vi "Cued Discrmination Tasks w PCO (Most Recent).vi"() -> ()   [LabVIEW 2015]
uses:
  <vilib>/Utility/error.llb/DialogType.ctl
  <vilib>/Platform/TimedLoop/XDataNode/timing_clust.ctl
  <vilib>/Platform/TimedLoop/XDataNode/nitl_modes.ctl
  <vilib>/Platform/TimedLoop/XDataNode/wakeup.ctl
  <vilib>/DAQmx/read.llb/DAQmx Read (Analog 1D DBL 1Chan NSamp).vi
  <vilib>/DAQmx/read.llb/DAQmx Read (Digital Wfm 1Chan NSamp).vi
  <vilib>/DAQmx/read.llb/DAQmx Read (Counter DBL 1Chan 1Samp).vi
  <vilib>/DAQmx/write.llb/DAQmx Write (Digital Bool 1Line 1Point).vi
  <vilib>/DAQmx/write.llb/DAQmx Write (Analog 2D DBL NChan NSamp).vi
  <vilib>/DAQmx/miscellaneous.llb/DAQmx Fill In Error Info.vi
  <vilib>/platform/TimedLoop/XDataNode/XDataNode.xnode
  <vilib>/Platform/TimedLoop/XDataNode/XDNodeRunTimeDep.lvlib
panel:
  out "Stim 2":i32
  out "False Alarm":bool
  out "Diag Start Time":u32
  out "Licked":bool
  out "Reward Start (ms) \n(Discrim Vary) 2":u32
  out "Stim Start Dist \n(Discrim Vary) 2":sgl
  out "Stim Start Time\n(Discrim Vary)  2":u32
  out "Stim\nReceived 2":bool
  out "Stim\nReceived":bool
  out "Stim":i32
  out "StimInfo":i32[](array[numeric])
  out "Vert\nVariant":bool=TRUE
  out "Small Stim":bool=TRUE
  out "Numeric":i32
  out "Stim Start Dist \n(Cue Only)":sgl
  out "Stim Start Time\n(Cue Only)":u32
  out "Reward Start (ms) \n(Cue Only)":u32
  out "Stim Start Time\n(Discrim Vary)":u32
  out "Stim Start Time\n(Discrim Only)":u32
  out "Stim Variation":i16
  out "Unity Info Q":refnum<queue>
  out "Unity Version Q":refnum<queue>
  out "Stim Start Dist \n(Discrim Vary)":sgl
  out "Lick Begin \n- RZ One  2":bool=TRUE
  out "Reward Start (ms) \n(Discrim Vary)":u32
  out "Varied Stim":string
  in  "Test Encoder Speed \n(Timed Loop Period)":i64=15
  in  "Test Encoder":bool
  out "Stim Identity":string
  out "Rand Number Created":bool=TRUE
  out "UDP test":i32
  out "Unity Stim Q":refnum<queue>
  in  "Stop Unity Receive":bool
  out "UDP error":errorcluster
  out "Total Dist Travelled":dbl
  out "Reward Start (ms) \n(Discrim Only)":u32
  out "Lick Begin \n- RZ One":bool=TRUE
  out "Stim Start Dist\n(Discrim Only)":sgl
  in  "Reward Zone Finish":sgl=70.0
  in  "Reward Zone Start":sgl=30.0
  out "Encoder Ref Out":refnum<file>
  out "Encoder Ref Error":errorcluster
  out "Timer Q Out":refnum<queue>
  out "Elapsed Time":dbl caption="Elapsed Time (s)"
  out "Encoder\n Ref Out 2":refnum<file>
  out "PCo Ref Error":errorcluster
  out "File Iterations":i32
  out "Save Start Time":dbl
  out "Save Time Start":bool=TRUE
  in  "Ignore PCO":bool=TRUE
  in  "SAVE":bool
  out "Reward Start (ms) - \nRun Train":u32
  in  "Droplet Duration":u32=150
  out "Lick Waveform":i16(graph)
  out "Correct":bool
  in  "Give Soymilk":bool
  in  "Distance \nTriggered":bool
  in  "Lick Window(ms)":u32=800
  out "File Save Path":path
  in  "MODE":T1(ring)
  in  "Reward\n Distance":dbl
  in  "Rand Stim\nDist Interval":dbl=150.0 format="%#_13g"
  in  "Stop Encoder":bool
  out "Relative \nRand Dist":dbl
  in  "Hot Pixel Corr":bool
  in  "Noise Filter":bool
  in  "Mouse Name":string
  out "Red Waveform":dbl(graph)
  in  "Stop Red Stamp":bool
  out "Red Q Out":refnum<queue>
  in  "NewTrial":bool
  out "Stim ref out 2":refnum<file>
  out "Eye Track Info":sgl[](array[numeric])
  out "Eye Track Q":refnum<queue>
  out "Eye It Q":refnum<queue>
  in  "Stop Eye Cam UDP":bool
  out "Eye Iterations":u32
  out "PCO iterations":u32
  in  "Close Trigger 2":bool
  in  "Port":u16=6342
  out "bClose":bool
  in  "TriggerMode":u16(ring)=2 items=["Auto", "Software", "External sequence start ", "External exposure control"]
  in  "Delay":u32
  in  "ExposureTimeBase":u16(ring)=2 items=["nanoseconds", "microseconds", "milliseconds"]
  in  "DelayTimeBase":u16(ring)=2 items=["nanoseconds", "microseconds", "milliseconds"]
  in  "ROIX0":u16=961 min=1
  in  "ROIY0":u16=811 min=1
  out "PCO Image":u16[][](graph)
  out "PCO Ref Out 2":refnum<file>
  out "bUseBuffer0":bool
  out "bUseBuffer1":bool
  in  "Pixel Rate":i32(ring) items=["286000000", "0", "0", "0"]
  in  "Exposure":dbl=50.0
  in  "ROIX1":u16=1600
  in  "ROIY1":u16=1350
  in  "UseAcquireEnable":bool
  out "PCO Recording":bool
  in  "Close PCO":bool
  out "Bits/pixel":u16
  out "BufNr1":i16
  out "BufNr0":i16
  out "Stim ref out":refnum<file>
  out "seed 7":dbl=74805.0
  in  "xcenter 10":i32=1800
  in  "xcenter 7":i32=1800
  out "seed 5":dbl=32848.0
  out "seed 4":dbl=8420.0
  out "seed  3":dbl=16239.0
  out "seed  1":dbl=85122.0
  in  "Start Stimulus":bool
  in  "Stop TCP Write":bool
  in  "frames to avg":i32=20
  in  "Tab Control":T2(tab)=enum."akmovingspotsII"
  in  "Stimlength (s)":dbl=1.0
  in  "Scaling factor":dbl=1.0
  in  "Rects per width":dbl=320.0
  in  "Rects per height":dbl=1.0
  in  "radius":dbl=4.0
  in  "interval (s)":dbl=0.5
  in  "# of circles":dbl=10.0
  in  "# of flashes/circles":dbl=10.0
  in  "ring width":dbl=4.0
  in  "interval 2 (ms)":dbl=500.0
  in  "# of flashes/ring":dbl=2.0
  in  "spot intensity":dbl=255.0
  in  "Velocity (pix/s)":dbl=100.0
  in  "Length (pixels)":dbl=40.0
  in  "Width (pixels)":dbl=1920.0
  in  "repeats 4":i32=4
  in  "Background\nangle":dbl
  in  "Background\ncycles/s":dbl=1.0
  in  "Background\nspatial frequency":dbl=0.05
  in  "Differential time":i32=2
  in  "Local time":i32=2
  in  "Global time":i32=2
  in  "Object angle":i32=180
  in  "Object size":i32=100
  in  "Object phase":dbl
  in  "radius 2":dbl=50.0
  in  "time interval (ms)":dbl=500.0
  in  "# of x spots":dbl=2.0
  in  "# of y spots":i32=2
  in  "# of flashes/spot":i32=1
  in  "repeats 9":i32=2
  in  "flash frame length 2":i32=8
  in  "# of flashes 2":i32=8
  in  "repeats 2":dbl
  in  "y velocity":dbl
  in  "x velocity":dbl
  in  "line width":dbl
  in  "cycles per second":i32=2
  in  "period":i32=200
  in  "duration":i32=8
  in  "repeats":i32=3
  in  "amplitude":i32=100
  in  "amplitude 3":i32=100
  in  "repeats 13":i32=3
  in  "duration 3":i32=6
  in  "period 3":i32=240
  in  "cycles per second 3":i32=2
  out "seed 2":dbl=28230.0
  in  "# of flashes":i32=8
  in  "flash frame length":i32=8
  in  "repeats  11":i32=3
  in  "flashnum":i32=1
  in  "msinterval 4":i32=500
  in  "chopy":i32=5
  in  "chopx":i32=5
  in  "grayframes":i32=30
  in  "flashbrightness":i32
  in  "boxsize":i32
  in  "xcenter 4":i32
  in  "ycenter 4":i32
  in  "ycenter 6":i32
  in  "xcenter 6":i32
  in  "boxsize 2":i32
  in  "flashbrightness 2":i32
  in  "grayframes 2":i32=30
  in  "repeats  12":i32=4
  in  "flashnum 2":i32=1
  in  "msinterval 5":i32=500
  in  "chopy 2":i32=10
  in  "chopx 2":i32=10
  in  "length":i32=40
  in  "pixels/frame":i32=4
  in  "width":i32=1960
  in  "repeats 11":i32=3
  in  "bardiv":i32=1
  in  "backg 2":i32=127
  in  "barbrightness":i32
  out "seed":dbl=11328.0
  in  "0 for 90, 1 for 45":i32
  in  "graydelayframes":i32=120
  in  "RFcentered=1":i32
  in  "xcenter 5":i32
  in  "ycenter 5":i32
  in  "ycenter 8":i32
  in  "xcenter 8":i32
  in  "RFcentered=1 2":i32
  in  "graydelayframes 3":i32=120
  in  "0 for 90, 1 for 46":i32=1
  out "seed  6":dbl=32848.0
  in  "barbrightness 3":i32
  in  "backg 4":i32=127
  in  "bardiv 3":i32=1
  in  "repeats 16":i32=25
  in  "width 3":i32=1960
  in  "length 3":i32=40
  in  "pixels/frame 3":i32=4
  in  "grayframes 3":dbl=10.0
  in  "repeats 17":dbl=10.0
  in  "width 4":dbl=40.0
  in  "bars":dbl=4.0
  in  "grayframes  4":dbl=240.0
  in  "repeats  19":dbl=8.0
  in  "width  5":dbl=40.0
  in  "bars  2":dbl=6.0
  in  "grayframes  5":dbl=240.0
  in  "repeats  20":dbl=8.0
  in  "width  6":dbl=40.0
  in  "bars  3":dbl=6.0
  in  "appatchsizelitude 6":i32=300
  in  "ycenter 7":i32=500
  in  "xcenter 9":i32=1500
  in  "amplitude 5":i32=100
  in  "repeats 15":i32=10
  in  "duration 6":i32=1
  in  "period 5":i32=300
  in  "cycles per second 5":i32=1
  out "seed 6":dbl=32105.0
  in  "asdf":i32=100
  in  "asdf 2":i32=3
  in  "numpatches":i32=5
  in  "amplitude 6":i32=100
  in  "repeats 19":i32=3
  in  "duration 7":i32=5
  in  "period 6":i32=80
  in  "cycles per second 6":i32=3
  out "randinput 5":dbl=10207.0
  in  "blanktime 2":dbl=8000.0
  in  "0 for bar \n1 for cross":dbl
  in  "backg 5":dbl=127.0
  in  "centery 2":dbl=650.0
  in  "centerx 2":dbl=1500.0
  in  "repeats 18":dbl=20.0
  in  "msinterval 6":dbl=12000.0
  in  "speed 2":dbl=1.0
  in  "bar radius":dbl=1500.0
  in  "graydelayframes 2":i32
  in  "degrees":i32
  out "seed  4":dbl=22949.0
  in  "barbrightness 2":i32
  in  "backg 3":i32=127
  in  "bardiv 2":i32=1
  in  "repeats 12":i32=2
  in  "width 2":i32=1960
  in  "length 2":i32=40
  in  "pixels/frame 2":i32=4
  out "randinput 2":dbl=74805.0
  in  "grayDelay":dbl=1000.0
  in  "msinterval 2":dbl=1000.0
  in  "msDelay":dbl=1000.0
  in  "initRadius":dbl=25.0
  in  "rate":dbl=4.0
  in  "repeats 6":dbl=1.0
  in  "ycenter 2":dbl=500.0
  in  "xcenter 2":dbl=1500.0
  out "randinput 4":dbl=28230.0
  in  "grayDelay 2":dbl=1000.0
  in  "msinterval 3":dbl=1000.0
  in  "msDelay 2":dbl=1000.0
  in  "initRadius 2":dbl=25.0
  in  "rate 2":dbl=4.0
  in  "repeats 10":dbl=1.0
  in  "ycenter 3":dbl=500.0
  in  "xcenter 3":dbl=1500.0
  in  "dycenter":dbl=1000.0
  in  "dxcenter":dbl=1000.0
  in  "offsetms":dbl=1000.0
  in  "backg":dbl=127.0
  in  "centery":dbl=500.0
  in  "centerx":dbl=1700.0
  in  "repeats 3":dbl=4.0
  in  "msinterval":dbl=1000.0
  in  "speed":dbl=10.0
  in  "ringR":dbl=4.0
  in  "bool":dbl=1.0
  in  "blanktime":dbl=6000.0
  out "randinput":dbl=12910.0
  in  "background 2":i32=127
  in  "ycenter":i32=500
  in  "radius 3":i32=250
  in  "rotation":i32=90
  in  "xcenter":dbl=1700.0
  in  "period in pixels":dbl=40.0
  in  "repeats 5":dbl=4.0
  in  "period 2":dbl=6000.0
  in  "increment":i32=25
  in  "duration 2":i32=6
  in  "radius 4":i32=150
  in  "repeats 7":dbl=4.0
  in  "Ycenter":dbl=500.0
  in  "Xcenter":dbl=1700.0
  in  "gridsize":i32=4
  in  "duration 4":dbl=2.0
  in  "repeats 8":dbl=5.0
  in  "1on 2off 3 onoff":dbl=1.0
  out "randinput 3":dbl=52142.0
  in  "spotsperflash":i32=2
  out "seed 3":dbl=74805.0
  in  "amplitude 4":i32=100
  in  "repeats 14":i32=3
  in  "duration 5":i32=5
  in  "period 4":i32=80
  in  "cycles per second 4":i32=3
  in  "Frequency":i32=3
  in  "Repeats":i32=80
  in  "startCue":i32=5
  in  "waitForDeviceStart":i32=5
  in  "beepLengthSecs":i32=5
  in  "beepPauseTime":i32=5
  in  "Frequency 2":i32=3
  in  "Repeats 2":i32=80
  in  "Loops":i32=5
  in  "beepLengthSecs 2":i32=5
  in  "beepPauseTime 2":i32=5
  in  "waitForDeviceStart  2":i32=5
  in  "startCue 2":i32=5
  out "Input Line":string="34 6 40 8 120 32848 200000 10000 -330795 -230833 1869660"
  out "TCP Loop\nRunning":bool
  out "TCP Listen\nStopped":bool
  out "yref":sgl=2.9999416
  out "xref":sgl=2.9999416
  out "zref":sgl=2.9999416
  out "number (0 to 1) 2":dbl=0.7615508373602138
  out "x position":sgl=-0.30801073
  out "y position":sgl=0.69161034
  out "z position":sgl=21.696537
  out "File Open":bool
  out "PCO ref out":refnum<file>
  in  "Close Save":bool
  # "For MultAlt audio pause time starts after first crinkle -- increase if needed"
  # "Cant have less than 40"
  # "Make sure File Open &\nSave All are OFF\n when starting the VI"
  # "Set to 15 during trials"
  # "Start Flea  --> Record PCO --> Start Scanbox or Unity --> Save Flea --> Save All --> Start Stim -- > Stop Save --> New Trial ON/OFF --> Start Save --> Start Stim"
  # "Set to \"External \nSequence Start\""
  # "set to 50"
  # "Rolling       Global \n\nROIX0            1               961      \nROIX1          650            1600\n\nROIY0            1                811\nROIY1          540             1350"
  # "leave \nunselected"
  # "Global\n                       Waveform\nExp.               FR         Trig Freq\n\n50      ms       10             20           \n40.36 ms       20             20\n33.3046 ms   30                      \n500 us         33.6 \n(min. exposure time)"
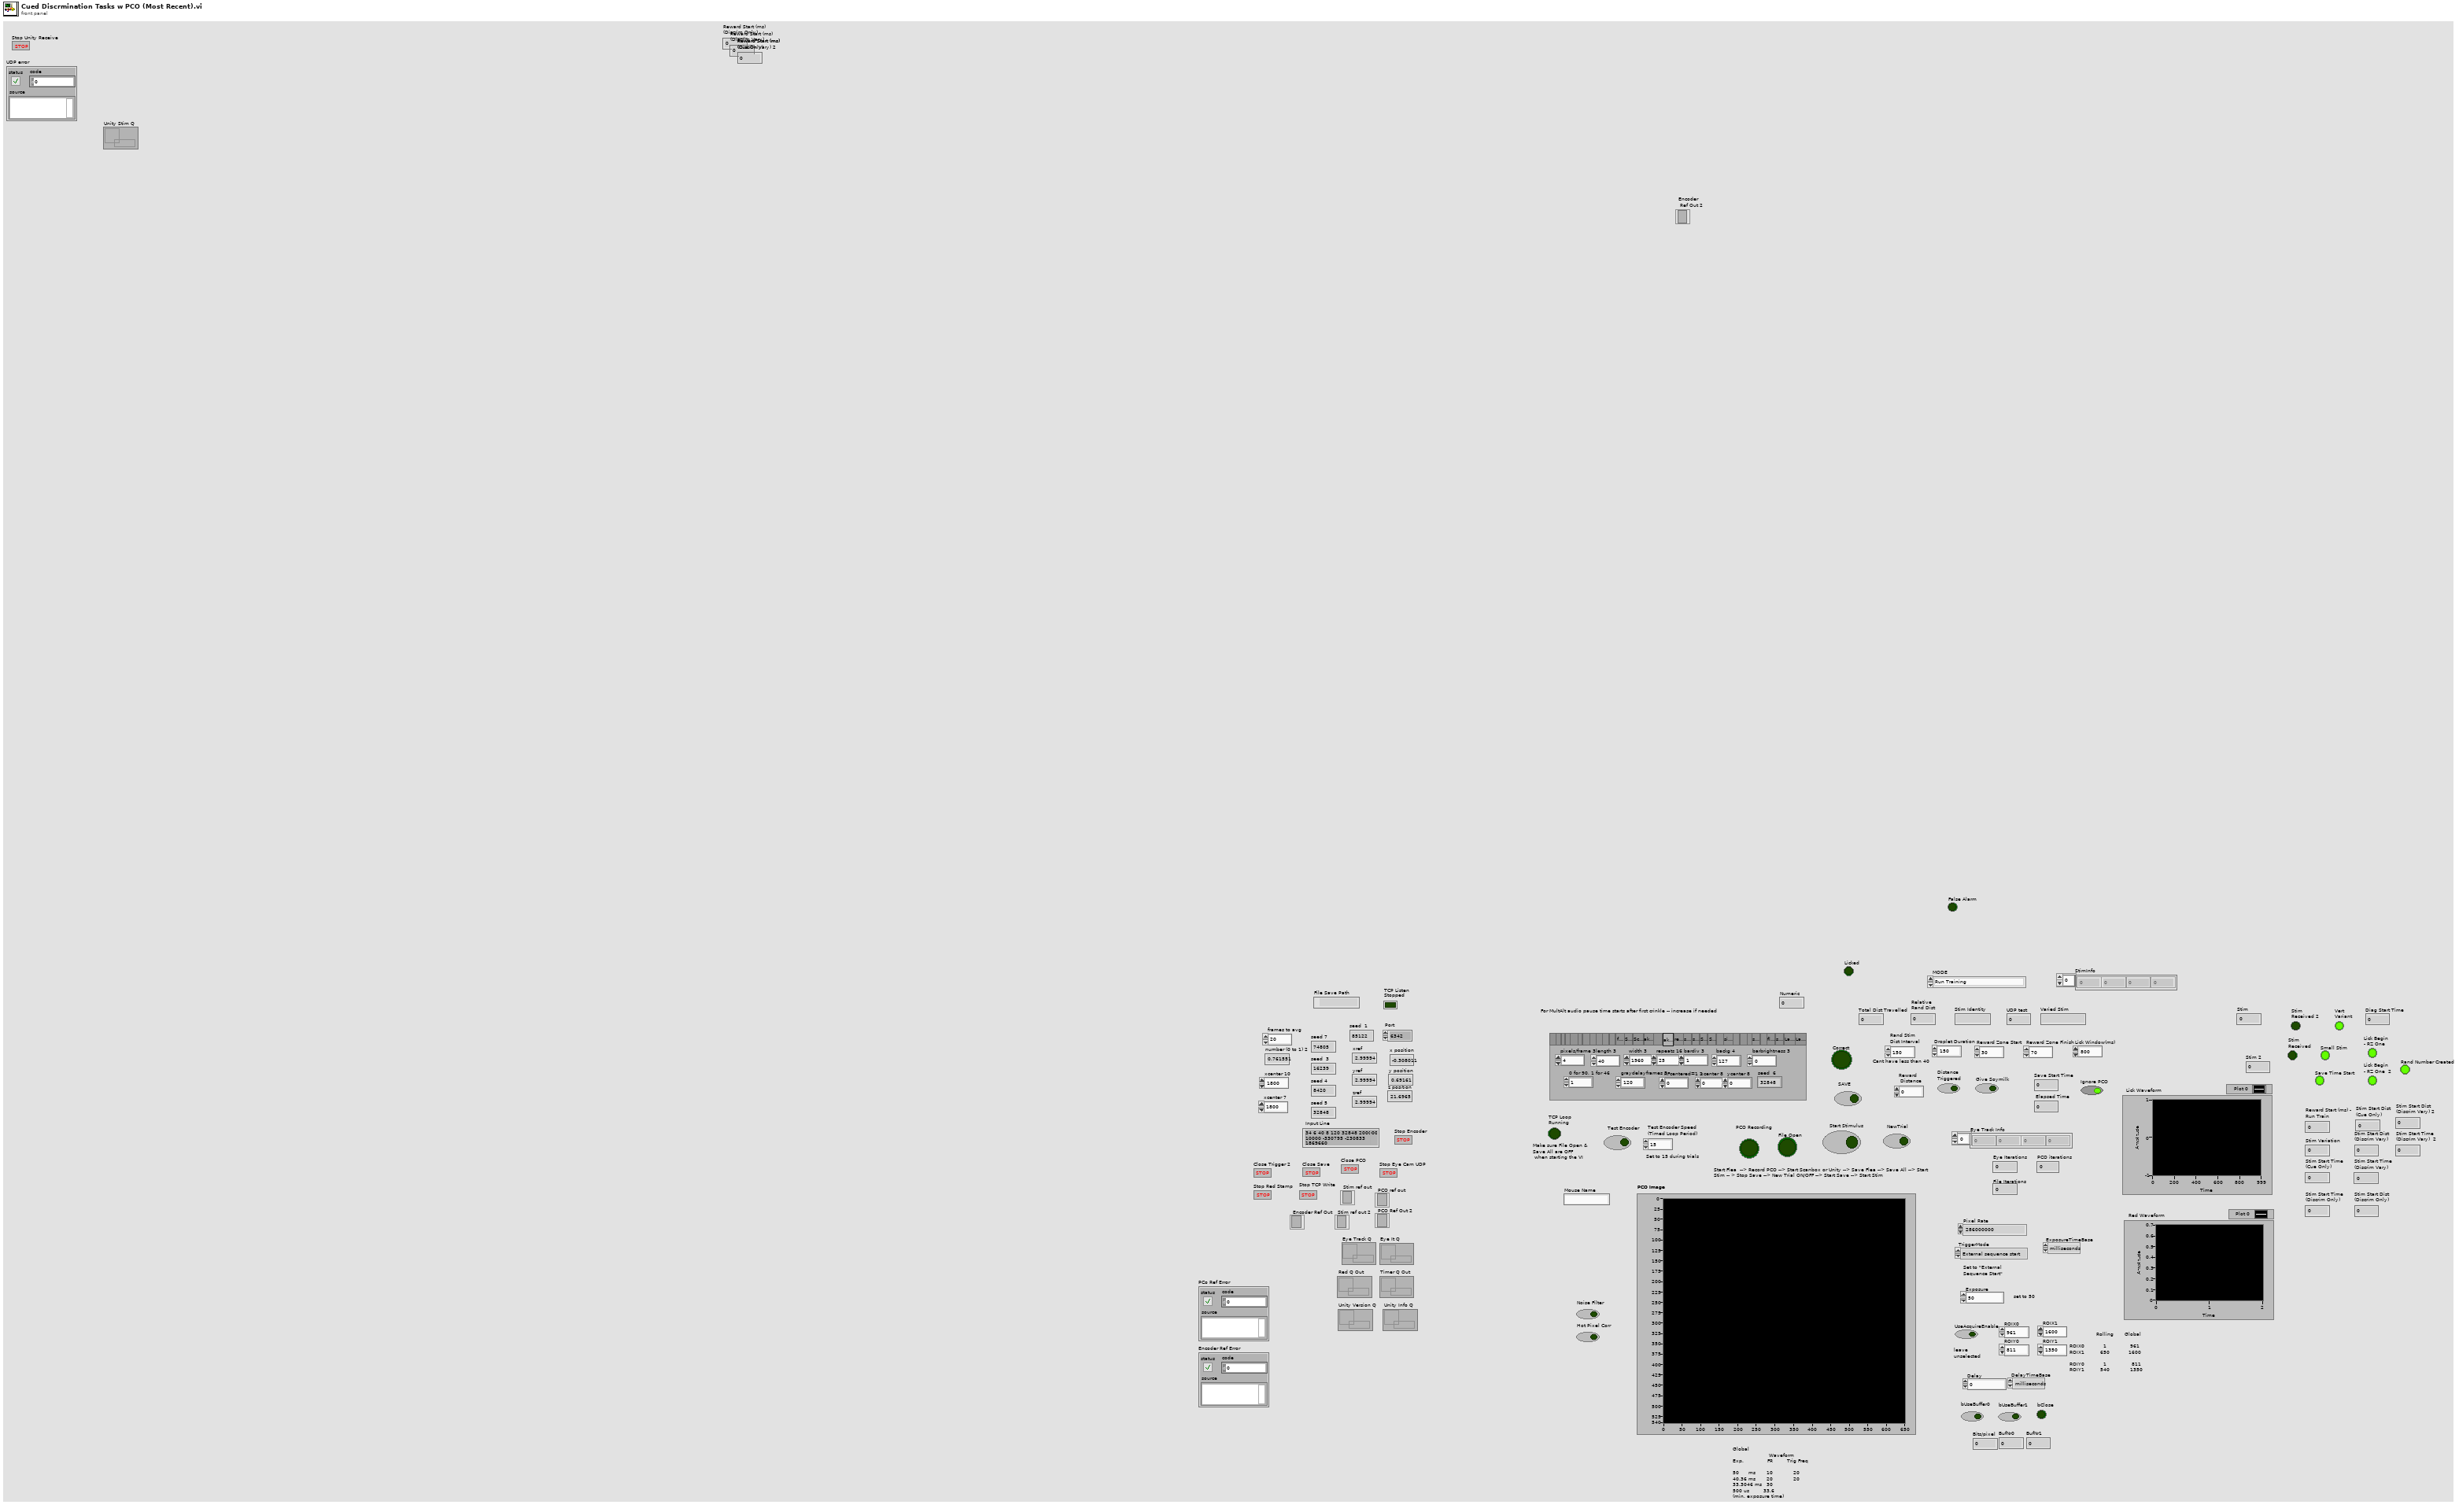
[diagram p1: front panel]
types:
  T1 = enum16{"Run Training", "Discrimination Only Task", "Discrimination Variant Task", "Alternating Variant Presentation", "Cued Attention Task "}
  T2 = enum32{"Barnoise", "Circle", "Ring", "Probe", "Moving bar", "OMS", "Rasterspot", "Fullfield", "whitebar", "driftgrat", "randgrat", "fullfieldonoff", "Screenchop", "Screenchopbars", "akmovingspots", "movingSpots", "akmovingspotsII", "retinotopybars", "slitGrtRand", "slitGrtOrder", "SqrGrtPtch", "SqrGrtPtch 2", "pinwheel", "singledirection", "newloom", "distractor", "loom", "switchgrate", "spotramp", "flickerspots", "squarewave", "LatCrinkleOneAlt", "LatCrinkleMultAlt"}
  T3 = typedef "DialogType.ctl" = u16
  T4 = cluster{"Size":u16, "CamType":u16, "CamSubType":u16, "SerialNumber":u32, "HWVersion":u32, "FWVersion":u32, "InterfaceType":u16, "HardwareVersion":cluster{"BoardNum":u16, "HWVersions":cluster{"BoardName":string, "BatchNumber":u16, "MinorRevision":u8, "MajorRevision":u8, "Variant":u16}[]}, "FirmwareVersion":cluster{"DeviceNum":u16, "FWVersions":cluster{"DeviceName":string, "MinorRevision":u8, "MajorRevision":u8, "Variant":u16}[]}}
  T5 = cluster{"Size":u16, "SensorTypeDESC":u16, "SensorSubtypeDESC":u16, "MaxHorizontalResStdDESC":u16, "MaxVerticalResStdDESC":u16, "MaxHorizontalResExtDESC":u16, "MaxVerticalResExtDESC":u16, "DynResDESC":u16, "MaxBinHorzDESC":u16, "BinHorzStepDESC":bool, "MaxBinVertDESC":u16, "BinVertStepDESC":bool, "ROIHorzStepDESC":u16, "ROIVertStepDESC":u16, "NumADCDESC":u16, "IRDESC":bool, "MinDelayDESC":u32, "MaxDelayDESC":u32, "MinDelayStepDESC":u32, "MinExpoDESC":u32, "MaxExpoDESC":u32, "MinExpoStepDESC":u32, "MinDelayIRDESC":u32, "MaxDelayIRDESC":u32, "MinExpoIRDESC":u32, "MaxExpoIRDESC":u32, "TimeTableDESC":bool, "DoubleImageDESC":bool, "MinCoolSetDESC":i16, "MaxCoolSetDESC":i16, "MDefaultCoolSetDESC":i16, "PowerDownModeDESC":bool, "OffsetRegDESC":bool, "ColorPattern":cluster{"UpperLeftColor":u8, "UpperRightColor":u8, "LowerLeftColor":u8, "LowerRightColor":u8}, "PatternTypeDESC":bool, "PixelRates":u32[], "CoversionFactors":u16[], "Reserved":u32[], "NoiseFilterCapable":bool, "HotPixelCapable":bool, "HotPixelWithNoiseFilter":bool, "ASCIITimeCapable":bool, "Extended Description":bool, "Get Extended":bool, "Reserved Flag 1":bool, "Reserved Flag 2":bool}
  T6 = typedef "XDNodeRunTimeDep.lvlib/timing_clust.ctl" = cluster{"Expected End [f-1]":u64, "Actual End [f-1]":u64, "Finished Late? [f-1]":bool, "Expected End [i-1]":u64, "Actual End [i-1]":u64, "Finished Late? [i-1]":bool, "Expected Start [i]":u64, "Actual Start [i]":u64, "Expected Start [f]":u64, "Actual Start [f]":u64, "Source Name":string, "Structure Name":string, "Period":i64, "Deadline":i64, "Offset":i64, "Start":i64, "Priority":i32, "Timeout":i32, "Mode":T7, "Wakeup Reason":T8, "Error":errorcluster, "Source Type":string, "Secondary Source Type":string, "Global End Time":u64, "Global Start Time":u64, "Frame Duration":u64, "Iteration Duration":u64, "Assigned CPU":i32, "I/O Scan Engine Mode":u32}
  T7 = typedef "XDNodeRunTimeDep.lvlib/nitl_modes.ctl" = enum32{"No Change", "Process missed periods, maintain original phase", "Discard missed periods, maintain original phase", "Process missed periods, ignore original phase", "Discard missed periods, ignore original phase"}
  T8 = typedef "XDNodeRunTimeDep.lvlib/wakeup.ctl" = enum32{"Normal", "Aborted", "Asynchronous wakeup", "Timing source error", "Timed loop error", "Timeout"}
  T9 = enum16{"open", "replace", "create", "open or create", "replace or create", "replace or create with confirmation"}
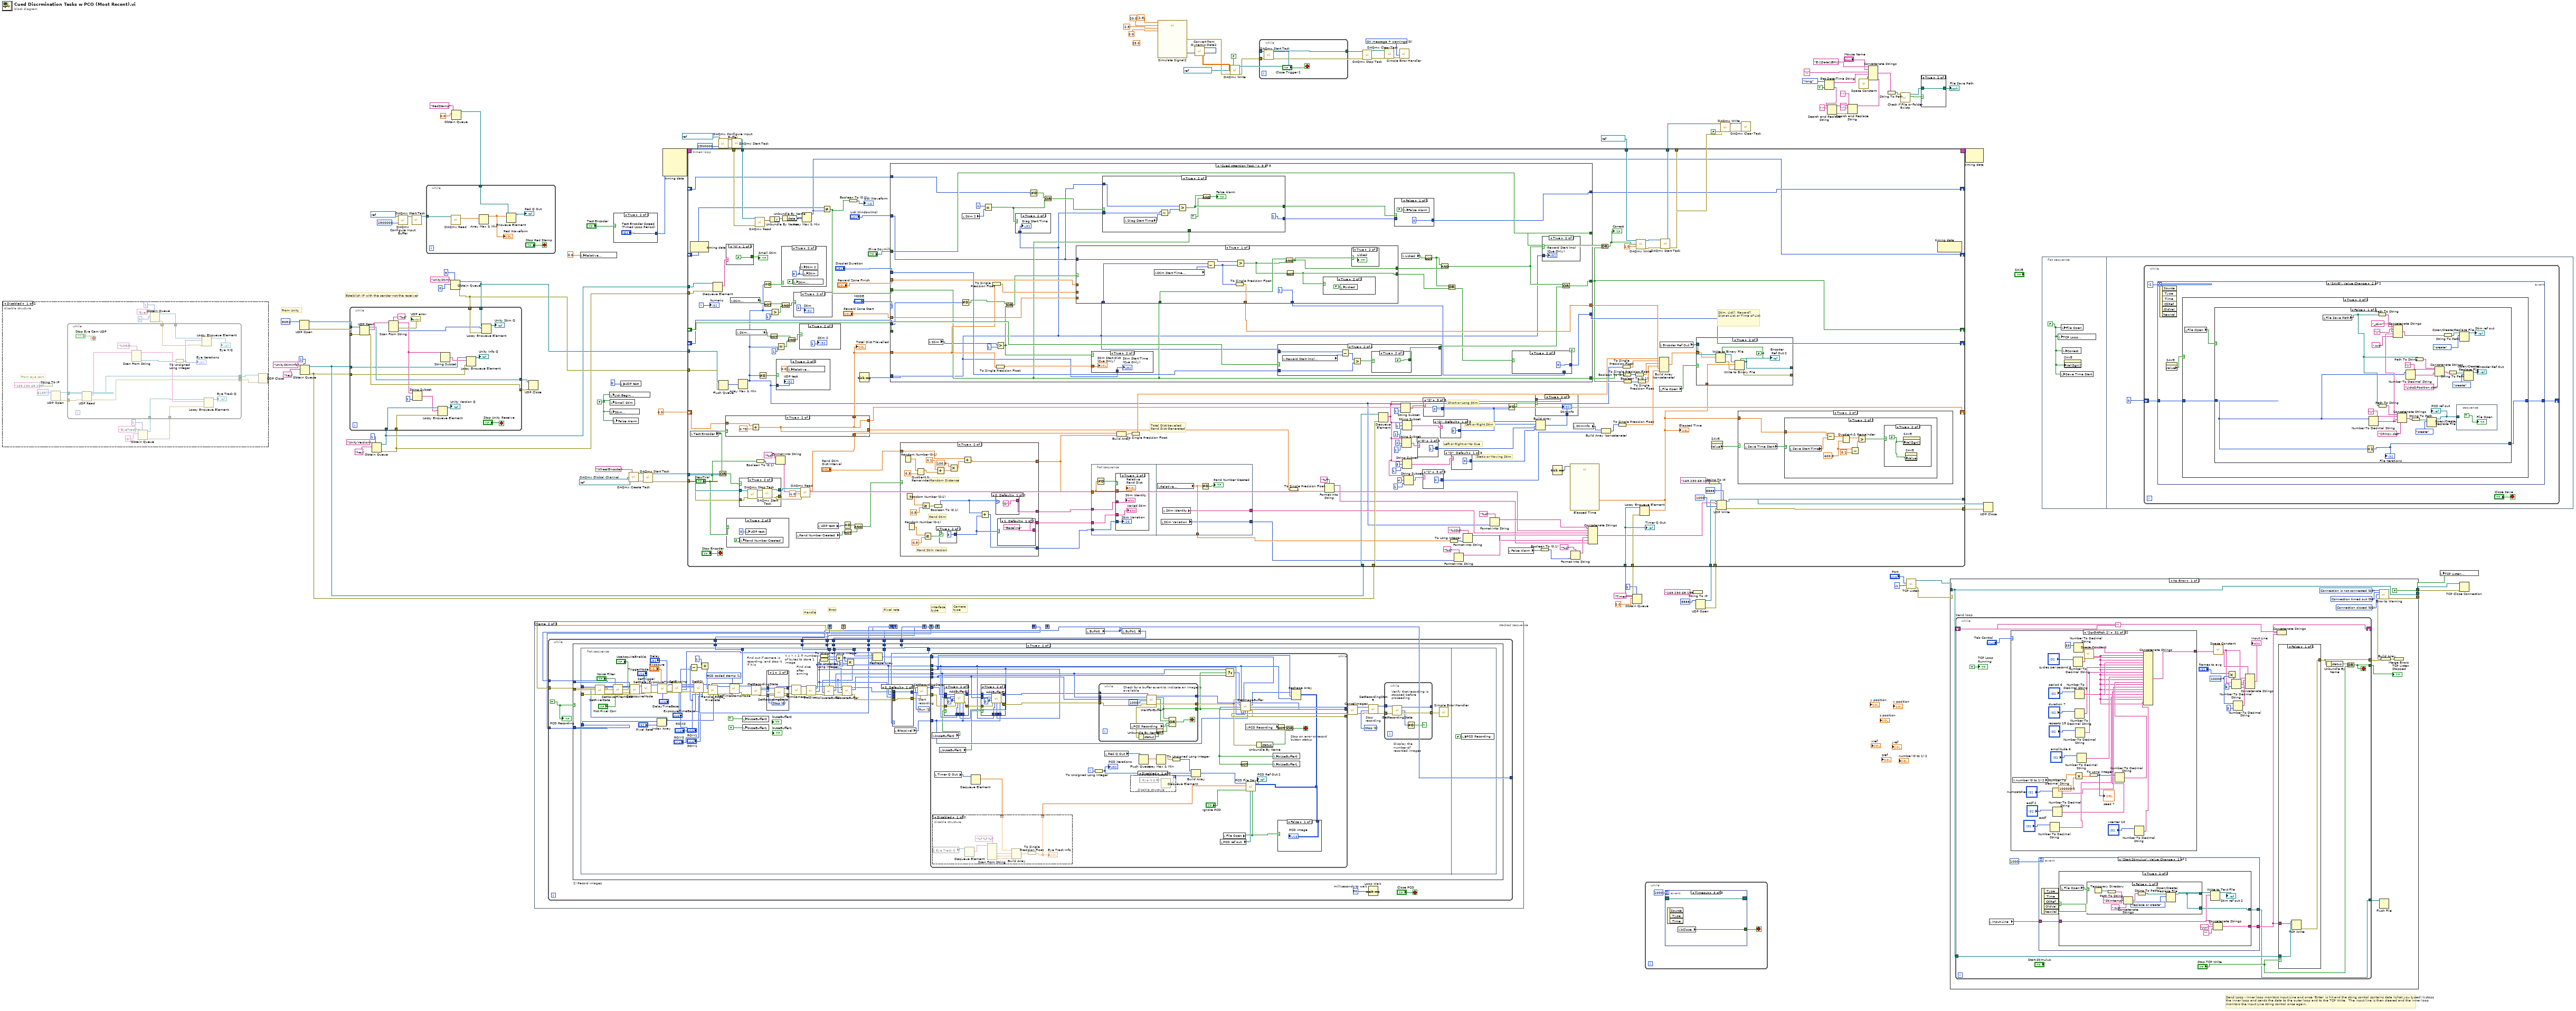
[diagram p0: block diagram]
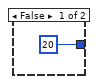
[diagram p3: hidden frame]
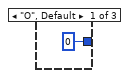
[diagram p4: hidden frame]
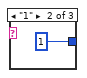
[diagram p5: hidden frame]
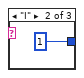
[diagram p10: hidden frame]
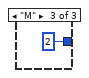
[diagram p11: hidden frame]
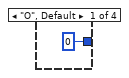
[diagram p12: hidden frame]
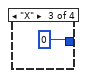
[diagram p13: hidden frame]
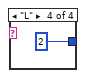
[diagram p14: hidden frame]
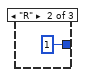
[diagram p15: hidden frame]
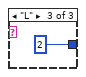
[diagram p16: hidden frame]
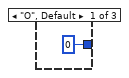
[diagram p17: hidden frame]
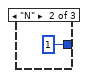
[diagram p18: hidden frame]
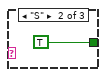
[diagram p19: hidden frame]
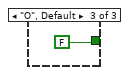
[diagram p20: hidden frame]
diagram:
  w1 = FALSE ("Lick Begin")
  w80 = refnum<k21> "MyLinearPositionChannel"  # DAQmx Global Channel
  (unwired) 25.0 ("Duty Cycle (%)")
  w97 = T3 3 items=["no dialog", "OK message", "continue or stop message", "OK message + warnings", "continue/stop + warnings"] ("type of dialog (OK msg:1)")
  # "From Unity"
  # "Establish IP with the sender not the receiver"
  # "Send Loop - Inner loop monitors Input Line and once 'Enter' is hit and the string control contains data (what you typed) it stops the inner loop and sends the data to the outer loop and to the TCP Write.  The input line is then cleared and the inner loop monitors the Input Line string control once again."
  # "Camera type"
  # "Interface type"
  # "Error"
  # "Handle"
  # "Pixel rate"
  n1 = disable-structure shown="Disabled" {
    frame Disabled {
      # "From eye cam"
      n2 = String To IP(1:"169.230.68.201" ("name")) -> ()  [unwired: 1 out]
      n3 = UDP Open(11:u16 61557 ("port")) -> (port=w121:refnum<k16>, 0:w118:errorcluster)  [unwired: 4 in, 1 out]
      n4 = Obtain Queue(max queue size (-1, unlimited)=1, name (unnamed)="EyeTrack", element data type="0" ("format string")) -> (queue out=w109:refnum<queue>, error out=w108:errorcluster)  [unwired: 2 in, 1 out]
      n5 = Obtain Queue(max queue size (-1, unlimited)=1, name (unnamed)="EyeIt", element data type=u32 0 ("Eye Iterations")) -> (queue out=w114:refnum<queue>, error out=w113:errorcluster)  [unwired: 2 in, 1 out]
      n6 = while {
        tunnel: w121 -> [w137]
        tunnel: [w135] -> w122
        tunnel: w118 -> [w136]
        tunnel: [w134] -> w123
        tunnel: w114 -> [w127]
        tunnel: w113 -> [w126]
        tunnel: w109 -> [w125]
        tunnel: w108 -> [w124]
        stop <- "Stop Eye Cam UDP" stop-if-true
        n7 = UDP Read(connection ID=w137, 8:w136) -> (data out=w129:string, error out=w134:errorcluster, 3:w135:refnum<k16>)  [unwired: 2 in, 2 out]
        n8 = Scan From String(format string="%05d", input string=w129) -> (remaining string=w128:string, output 1=w139:i32)  [unwired: 3 in, 2 out]
        n9 = To Unsigned Long Integer(number=w139) -> (unsigned 32bit integer=w133:u32)
        "Eye Iterations" <- w133
        n10 = Lossy Enqueue Element(queue=w127, element=w133, error in (no error)=w126) -> (queue out=→"Eye It Q":refnum<queue>)  [unwired: 3 out]
        n11 = Lossy Enqueue Element(queue=w125, element=w128, error in (no error)=w124) -> (queue out=→"Eye Track Q":refnum<queue>)  [unwired: 3 out]
      }
      n12 = UDP Close(connection ID=w122, 8:w123) -> ()  [unwired: 2 out]
    }
    frame Enabled {
    }
  }
  n13 = UDP Open(11:u16 8051 ("port")) -> (port=w24:refnum<k16>, 0:w23:errorcluster)  [unwired: 4 in, 1 out]
  n14 = Obtain Queue(max queue size (-1, unlimited)=1, name (unnamed)="UnityStimInfo", element data type="hey") -> (queue out=w4:refnum<queue>, error out=w3:errorcluster)  [unwired: 2 in, 1 out]
  n15 = Obtain Queue(max queue size (-1, unlimited)=1, name (unnamed)="UnityVersion", element data type="hey") -> (queue out=w8:refnum<queue>, error out=w7:errorcluster)  [unwired: 2 in, 1 out]
  n16 = call <vilib>:"DAQmx Configure Input Buffer.vi"("task/channels in"=refnum<k21> "RedStamp", "buffer size (in samples per channel)"=u32 2500000) -> ("task out"=w76:refnum<k21>)  [unwired: 12 in, 1 out]
  n17 = call <vilib>:"DAQmx Start Task.vi"("task/channels in"=w76) -> ("task out"=w78:refnum<k21>)  [unwired: 13 in, 1 out]
  n18 = Obtain Queue(max queue size (-1, unlimited)=5, name (unnamed)="UnityStim", element data type=0 ("Eye Iterations")) -> (queue out=w17:refnum<queue>, error out=w16:errorcluster)  [unwired: 2 in, 1 out]
  n19 = while {
    tunnel: w24 -> [w161]
    tunnel: w23 -> [w160]
    tunnel: [w150] -> w22
    tunnel: [w158] -> w21
    tunnel: w17 -> [w156]
    tunnel: w16 -> [w155]
    tunnel: w7 -> [w148]
    tunnel: w8 -> [w149]
    tunnel: w4 -> [w141]
    tunnel: w3 -> [w140]
    stop <- "Stop Unity Receive" stop-if-true
    n20 = UDP Read(connection ID=w161, 8:w160) -> (data out=w157:string, error out=w158:errorcluster, 3:w150:refnum<k16>)  [unwired: 2 in, 2 out]
    n21 = Scan From String "Scan From String"(format string="%d", input string=w157) -> (remaining string=w144:string, error out=→"UDP error":errorcluster, output 1=w154:i32)  [unwired: 3 in, 1 out]
    n22 = String Subset(string=w144, length (rest)=1 ("length (rest)")) -> (substring=w145:string)  [unwired: 1 in]
    n23 = Lossy Enqueue Element(queue=w149, element=w145, error in (no error)=w148) -> (queue out=→"Unity Version Q":refnum<queue>)  [unwired: 3 out]
    n24 = String Subset(string=w144) -> (substring=w142:string)  [unwired: 2 in]
    n25 = Lossy Enqueue Element(queue=w141, element=w142, error in (no error)=w140) -> (queue out=→"Unity Info Q":refnum<queue>)  [unwired: 3 out]
    n26 = Lossy Enqueue Element(queue=w156, element=w154, error in (no error)=w155) -> (queue out=→"Unity Stim Q":refnum<queue>)  [unwired: 3 out]
  }
  n27 = Obtain Queue(name (unnamed)="RedStamp", element data type=0.0 ("max value")) -> (queue out=w74:refnum<queue>)  [unwired: 3 in, 2 out]
  n28 = while {
    tunnel: w78 -> [w167]
    tunnel: w74 -> [w165]
    stop <- "Stop Red Stamp" stop-if-true
    n29 = call-poly <vilib>:"DAQmx Read.vi"("task/channels in"=w167) -> ("data"=w163:dbl[])  [unwired: 12 in, 2 out]
    n30 = Array Max & Min(array=w163) -> (max value=w162:dbl)  [unwired: 3 out]
    "Red Waveform" <- w162
    n31 = Enqueue Element(queue=w165, element=w162) -> (queue out=→"Red Q Out":refnum<queue>)  [unwired: 2 in, 2 out]
  }
  n32 = UDP Close(connection ID=w22, 8:w21) -> ()  [unwired: 2 out]
  n33 = stacked-sequence {
    seq-local: [w212 _ _] -> [_ w232 _]
    seq-local: [w185 _ _] -> [_ _ _]
    seq-local: [w173 _ _] -> [_ w235 w456]
    seq-local: [w174 _ _] -> [_ w234 w455]
    seq-local: [w210 _ _] -> [_ w233 _]
    seq-local: [w200 _ _] -> [_ w229 _]
    seq-local: [w187 _ _] -> [_ w228 _]
    seq-local: [w184 _ _] -> [_ w227 _]
    seq-local: [w183 _ _] -> [_ w226 _]
    frame #0 {
      w202 = FALSE ("stop")
      # "Setup greyscale palette for intensity graph display: Color = i*(0x01 + 0x100 + 0x10000)"
      # "1) Setup camera"
      # "Find out if camera uses CameraLink"
      # "Initialize a LabVIEW array of X x Y integers to hold image"
      # "Open communication with a camera and find its properties"
      n34 = local write "PCO Recording"(w202) -> ()
      n35 = local write "bClose"(w202) -> ()
      n36 = call <vilib>:"Reset_SDK_Lib.vi"() -> ("ErrorOut"=w168:errorcluster)  [unwired: 11 in]
      n37 = call <vilib>:"OpenCamera.vi"("ErrorIn"=w168) -> ("ErrorOut"=w198:errorcluster, "Handle out"=w199:u64)  [unwired: 3 in, 2 out]
      n38 = call <vilib>:"InitLibrary.vi"("error in (no error)"=w198, "InterfaceType"=u32 3, "ph"=w199) -> ("error out"=w197:errorcluster, "hout"=w196:u64)  [unwired: 7 in]
      n39 = for {
        N: 256 -> [_]
        tunnel: [w216] -> w178 mode=indexing
        i -> [w217]
        n40 = Multiply(x=65793, y=w217) -> (x*y=w216:i32)
      }
      n41 = call <vilib>:"GetCameraType.vi"("ph"=w196, "error in (no error)"=w197) -> ("hout"=w182:u64, "CameraType"=w188:T4, "error out"=w181:errorcluster)  [unwired: 1 in, 1 out]
      n42 = call <vilib>:"GetDescription.vi"("ErrorIn"=w181, "ph"=w182) -> ("ErrorOut"=w170:errorcluster, "Description"=w211:T5, "hout"=w172:u64)  [unwired: 2 in, 1 out]
      n43 = call <vilib>:"GetAcquireEnableSignalStatus.vi"("error in (no error)"=w170, "ph"=w172) -> ("error out"=w169:errorcluster, "hout"=w171:u64)  [unwired: 2 in, 2 out]
      n44 = Unbundle By Name(w188) -> ("InterfaceType"=w210:u16)
      n45 = Unbundle By Name(w188) -> ("CamType"=w187:u16)
      n46 = property on="PCO Image" class="IntGraph (strict)"("Y Scale.Flipped"=TRUE, "X Scale.Flipped"=FALSE, "Color Table"=w178) -> ()  [unwired: 2 in, 2 out]
      n47 = Unbundle By Name(w211) -> ("DynResDESC"=→"Bits/pixel":u16, "PixelRates"=w200:u32[], "MaxHorizontalResStdDESC"=w176:u16, "MaxVerticalResStdDESC"=w175:u16, "MaxBinHorzDESC"=w184:u16, "MaxBinVertDESC"=w183:u16)  [unwired: 4 out]
      n48 = Number To Decimal String(number=w200) -> (decimal integer string=w201:string[])  [unwired: 1 in]
      n49 = property on="Pixel Rate" class="Ring (strict)"("Strings []"=w201) -> ()  [unwired: 2 in, 2 out]
      n50 = call <vilib>:"GetRecordingState.vi"("ErrorIn"=w169, "ph"=w171) -> ("ErrorOut"=w192:errorcluster, "Error"=w186:i32, "hout"=w193:u64)  [unwired: 2 in, 1 out]
      n51 = To Unsigned Long Integer(number=w176) -> (unsigned 32bit integer=w207:u32)
      n52 = To Unsigned Long Integer(number=w175) -> (unsigned 32bit integer=w206:u32)
      n53 = case shown="0, Default" w186 {
        tunnel: w193 -> [w222 w225]
        tunnel: w192 -> [w221 w224]
        tunnel: [w220 w225] -> w191
        tunnel: [w219 w224] -> w189
        frame 0, Default {
          w223 = u16 0 items=["Stop", "Run"] ("RecordingState")
          n54 = call <vilib>:"SetRecordingState.vi"("ErrorIn"=w221, "RecordingState"=w223, "ph"=w222) -> ("ErrorOut"=w219:errorcluster, "hout"=w220:u64)  [unwired: 2 in, 1 out]
        }
        frame 1 {
        }
      }
      n55 = Multiply(x=w207, y=w206) -> (x*y=w213:u32)
      n56 = Initialize Array(u16 0 ("Element Data"), w213) -> (w212:u16[])
      n57 = Multiply(x=w213, y=u32 2) -> (x*y=w185:u32)
      n58 = call <vilib>:"AllocateBuffer.vi"("error in (no error)"=w189, "Size"=w185, "BufNr"=i16 -1, "ph"=w191) -> ("error out"=w194:errorcluster, "BufNrOut"=→"BufNr0":i16, "hout"=w190:u64)  [unwired: 2 in, 3 out]
      n59 = call <vilib>:"AllocateBuffer.vi"("error in (no error)"=w194, "BufNr"=i16 -1, "ph"=w190) -> ("error out"=w174:errorcluster, "BufNrOut"=→"BufNr1":i16, "hout"=w173:u64)  [unwired: 3 in, 3 out]
    }
    frame #1 {
      n60 = local read "BufNr0"() -> (w231:i16)
      n61 = local read "BufNr1"() -> (w230:i16)
      n62 = while {
        tunnel: w231 -> [_]
        tunnel: w231 -> [w244]
        tunnel: w232 -> [w246]
        tunnel: w233 -> [w247]
        tunnel: w234 -> [w245]
        tunnel: w235 -> [w242]
        tunnel: w230 -> [w243]
        tunnel: w229 -> [w241]
        tunnel: w228 -> [w240]
        tunnel: w227 -> [w239]
        tunnel: w226 -> [w238]
        stop <- "Close PCO" stop-if-true
        w236 = TRUE
        w248 = u32 50  # milliseconds to wait
        n63 = case "2) Record images" shown="True" w236 {
          tunnel: w242 -> [_ w258]
          tunnel: w245 -> [_ w257]
          tunnel: w247 -> [_ w256]
          tunnel: w246 -> [_ w255]
          tunnel: w244 -> [_ w254]
          tunnel: w243 -> [_ w253]
          tunnel: w241 -> [_ w252]
          tunnel: w240 -> [_ w251]
          tunnel: w239 -> [_ w250]
          tunnel: w238 -> [_ w249]
          frame False {
          }
          frame True {
            n64 = flat-sequence {
              tunnel: w258 -> [w330]
              tunnel: w257 -> [w329]
              tunnel: w256 -> [w327]
              tunnel: w255 -> [w325]
              tunnel: w254 -> [w317]
              tunnel: w253 -> [w314]
              tunnel: w252 -> [w305]
              tunnel: w251 -> [w300]
              tunnel: w250 -> [w295]
              tunnel: w249 -> [w294]
              frame #0 {
                w271 = u16 1 items=["No time stamp", "BCD coded stamp", "BCD stamp + ASCII text"] ("TimeStampMode")
                w340 = u16 1 items=["Stop", "Run"] ("RecordingState")
                w343 = u16 0 items=["Stop", "Run"] ("RecordingState")
                # "Display the number of recorded images"
                # "Start recording"
                # "Find size after arming"
                # "Find out if camera is recording, and stop it if it is"
                # "X x Y x 2 = number of bytes to store 1 image"
                # "Stop recording"
                n65 = Index Array(array=w305, index="Pixel Rate") -> (element=w304:u32)
                n66 = call <vilib>:"SetPixelRate.vi"("error in (no error)"=w329, "PixelRate"=w304, "ph"=w330) -> ("error out"=w268:errorcluster, "hout"=w270:u64)  [unwired: 2 in, 1 out]
                n67 = call <vilib>:"SetNoiseFilterMode.vi"("error in (no error)"=w268, "Hot Pixel Corr"="Hot Pixel Corr", "Noise Filter"="Noise Filter", "ph"=w270) -> ("error out"=w267:errorcluster, "hout"=w269:u64)  [unwired: 1 out]
                n68 = call <vilib>:"SetAcquireMode.vi"("error in (no error)"=w267, "UseAcquireEnable"="UseAcquireEnable", "ph"=w269) -> ("error out"=w273:errorcluster, "hout"=w274:u64)  [unwired: 2 in, 1 out]
                n69 = call <vilib>:"SetTrigger.vi"("error in (no error)"=w273, "TriggerMode"="TriggerMode", "ph"=w274) -> ("error out"=w276:errorcluster, "hout"=w275:u64)  [unwired: 2 in, 1 out]
                n70 = call <vilib>:"SetDelayExposureTime.vi"("ph"=w275, "Delay"="Delay", "Exposure"="Exposure", "error in (no error)"=w276, "DelayTimeBase"="DelayTimeBase", "ExposureTimeBase"="ExposureTimeBase") -> ("hout"=w292:u64, "error out"=w291:errorcluster)  [unwired: 7 in, 1 out]
                n71 = call <vilib>:"SetBinning.vi"("error in (no error)"=w291, "BinVert"=w294, "BinHorz"=w295, "ph"=w292) -> ("error out"=w287:errorcluster, "hout"=w289:u64)  [unwired: 3 in, 1 out]
                n72 = Subtract(x="ROIX1", y="ROIX0") -> (x-y=w303:u16)
                n73 = call <vilib>:"SetROI.vi"("ph"=w289, "ROIX0"="ROIX0", "ROIY0"="ROIY0", "ROIX1"="ROIX1", "ROIY1"="ROIY1", "error in (no error)"=w287) -> ("hout"=w288:u64, "error out"=w286:errorcluster)  [unwired: 12 in]
                n74 = Add(x=1, y=w303) -> (x+y=w301:i32)
                n75 = call <vilib>:"Handle_Edge_Pixelrate.vi"("Cameratype"=w300, "error in (no error)"=w286, "PixelRate"=w304, "X-Resolution"=w301, "ph"=w288) -> ("error out"=w263:errorcluster, "hout"=w264:u64)  [unwired: 5 in]
                n76 = call <vilib>:"SetTimeStampMode.vi"("error in (no error)"=w263, "TimeStampMode"=w271, "ph"=w264) -> ("error out"=w260:errorcluster, "hout"=w259:u64)  [unwired: 1 out]
                n77 = local write "bUseBuffer0"(TRUE) -> ()
                n78 = local write "bUseBuffer1"(TRUE) -> ()
                n79 = call <vilib>:"GetRecordingState.vi"("ErrorIn"=w260, "ph"=w259) -> ("ErrorOut"=w337:errorcluster, "RecordingState"=w339:u16, "hout"=w338:u64)  [unwired: 2 in, 1 out]
                n80 = case shown="1" w339 {
                  tunnel: w338 -> [w448 w452]
                  tunnel: w337 -> [w447 w451]
                  tunnel: [w448 w450] -> w336
                  tunnel: [w447 w449] -> w335
                  frame 0, Default {
                  }
                  frame 1 {
                    w453 = u16 0 items=["Stop", "Run"] ("RecordingState")
                    n81 = call <vilib>:"SetRecordingState.vi"("ErrorIn"=w451, "RecordingState"=w453, "ph"=w452) -> ("ErrorOut"=w449:errorcluster, "hout"=w450:u64)  [unwired: 2 in, 1 out]
                  }
                }
                n82 = call <vilib>:"ArmCamera.vi"("error in (no error)"=w335, "ph"=w336) -> ("error out"=w261:errorcluster, "hout"=w262:u64)  [unwired: 1 in, 1 out]
                n83 = call <vilib>:"GetSizes.vi"("ph"=w262, "ErrorIn"=w261) -> ("hout"=w298:u64, "XResAct"=w323:u16, "YResAct"=w322:u16, "ErrorOut"=w297:errorcluster)  [unwired: 11 in, 3 out]
                n84 = To Unsigned Long Integer(number=w323) -> (unsigned 32bit integer=w318:u32)
                n85 = To Unsigned Long Integer(number=w322) -> (unsigned 32bit integer=w319:u32)
                n86 = Multiply(x=w318, y=w319) -> (x*y=w320:u32)
                n87 = Multiply(x=w320, y=u32 2) -> (x*y=w285:u32)
                n88 = call <vilib>:"AllocateBuffer.vi"("error in (no error)"=w297, "Size"=w285, "BufNr"=w317, "ph"=w298) -> ("error out"=w316:errorcluster, "BufNrOut"=w299:i16, "hout"=w315:u64)  [unwired: 2 in, 3 out]
                n89 = call <vilib>:"AllocateBuffer.vi"("error in (no error)"=w316, "Size"=w285, "BufNr"=w314, "ph"=w315) -> ("error out"=w283:errorcluster, "BufNrOut"=w313:i16, "hout"=w284:u64)  [unwired: 2 in, 3 out]
                n90 = Reshape Array(w325, w320) -> (w324:u16[])
                n91 = case shown="0, Default" w327 {
                  tunnel: [w440 w446] -> w331
                  tunnel: w322 -> [_ w445]
                  tunnel: w323 -> [_ w444]
                  tunnel: w284 -> [w440 w443]
                  tunnel: w283 -> [w439 w442]
                  tunnel: [w439 w441] -> w296
                  frame 0, Default {
                  }
                  frame 2 {
                    # "Only necessary if the interface is Camera Link"
                    n92 = call <vilib>:"CamLinkSetImageParameters.vi"("error in (no error)"=w442, "YRes"=w445, "XRes"=w444, "ph"=w443) -> ("error out"=w441:errorcluster, "hout"=w446:u64)  [unwired: 1 out]
                  }
                }
                n93 = local read "Bits/pixel"() -> (w310:u16)
                n94 = call <vilib>:"SetRecordingState.vi"("ErrorIn"=w296, "RecordingState"=w340, "ph"=w331) -> ("ErrorOut"=w328:errorcluster, "hout"=w326:u64)  [unwired: 2 in, 1 out]
                n95 = while {
                  tunnel: w299 -> [w380]
                  tunnel: w324 -> [w364]
                  tunnel: w326 -> [w384]
                  tunnel: w322 -> [w370]
                  tunnel: w323 -> [w368]
                  tunnel: w328 -> [w382]
                  tunnel: [w366] -> w309
                  tunnel: [w365] -> w308
                  tunnel: w313 -> [w373]
                  tunnel: w310 -> [w369]
                  i -> [w374]
                  stop <- w375 stop-if-true
                  # "Stop on error or record button status"
                  n96 = local read "bUseBuffer0"() -> (w359:bool)
                  n97 = local read "Timer Q Out"() -> (w345:refnum<queue>)
                  n98 = local read "bUseBuffer1"() -> (w358:bool)
                  n99 = case shown="True" w359 {
                    tunnel: [w399 w408] -> w381
                    tunnel: [w398 w407] -> w383
                    tunnel: w380 -> [_ w406]
                    tunnel: w384 -> [w398 w405]
                    tunnel: w369 -> [_ w403]
                    tunnel: w368 -> [_ w402]
                    tunnel: w370 -> [_ w401]
                    tunnel: w382 -> [w399 w400]
                    frame False {
                    }
                    frame True {
                      w404 = i16 0
                      n100 = call <vilib>:"AddBufferEX.vi"("ph"=w405, "BuffNr"=w406, "1stImage"=w404, "LastImage"=w404, "error in (no error)"=w400, "XRes"=w402, "YRes"=w401, "BitPerPixel"=w403) -> ("hout"=w407:u64, "error out"=w408:errorcluster)  [unwired: 5 in, 1 out]
                    }
                  }
                  n101 = Dequeue Element(queue=w345) -> (element=w344:dbl)  [unwired: 2 in, 3 out]
                  n102 = disable-structure shown="Disabled" {
                    disable-tunnel: [w389 _] -> w347
                    disable-tunnel: w344 -> [w388 _]
                    frame Disabled {
                      n103 = local read "Eye Track Q"() -> (w390:refnum<queue>)
                      n104 = Dequeue Element(queue=w390) -> (element=w395:string)  [unwired: 2 in, 3 out]
                      n105 = Scan From String(format string="%f %f %f", input string=w395) -> (output 1=w394:dbl, output 2=w393:dbl, output 3=w392:dbl)  [unwired: 5 in, 3 out]
                      n106 = Build Array(w388, w394, w393, w392) -> (w391:dbl[])
                      n107 = To Single Precision Float(number=w391) -> (single precision float=w389:sgl[])
                      "Eye Track Info" <- w389
                    }
                    frame Enabled {
                    }
                  }
                  n108 = case shown="True" w358 {
                    tunnel: [w409 w419] -> w371
                    tunnel: [w410 w418] -> w372
                    tunnel: w373 -> [_ w417]
                    tunnel: w383 -> [w410 w416]
                    tunnel: w369 -> [_ w414]
                    tunnel: w368 -> [_ w413]
                    tunnel: w370 -> [_ w412]
                    tunnel: w381 -> [w409 w411]
                    frame False {
                    }
                    frame True {
                      w415 = i16 0
                      n109 = call <vilib>:"AddBufferEX.vi"("ph"=w416, "BuffNr"=w417, "1stImage"=w415, "LastImage"=w415, "error in (no error)"=w411, "XRes"=w413, "YRes"=w412, "BitPerPixel"=w414) -> ("hout"=w418:u64, "error out"=w419:errorcluster)  [unwired: 5 in, 1 out]
                    }
                  }
                  n110 = To Unsigned Long Integer(number=w374) -> (unsigned 32bit integer=w352:u32)
                  "PCO iterations" <- w352
                  n111 = while {
                    tunnel: w380 -> [w421]
                    tunnel: [w431] -> w379
                    tunnel: [w429] -> w378
                    tunnel: [w427] -> w361
                    tunnel: w372 -> [w426]
                    tunnel: w371 -> [w425]
                    tunnel: w373 -> [w420]
                    stop <- w432 stop-if-true
                    # "Check for a buffer event to indicate an image is available"
                    n112 = local read "PCO Recording"() -> (w423:bool)
                    n113 = call <vilib>:"WaitForBuffer.vi"("ph"=w426, "sBufNr"=w421, "sBufNr 2"=w420, "timeout"=1000, "error in (no error)"=w425) -> ("hout"=w431:u64, "Buffer_Ready"=w427:bool, "Buffer_Ready 2"=w422:bool, "error out"=w429:errorcluster)  [unwired: 10 in, 1 out]
                    n114 = Unbundle By Name(w429) -> ("status"=w428:bool)
                    n115 = Not(x=w428) -> (.not. x?=w424:bool)
                    n116 = Compound Arithmetic op=OR(w427, w422, w423, w424) -> (w432:bool)
                  }
                  n117 = local read "Red Q Out"() -> (w355:refnum<queue>)
                  n118 = disable-structure shown="Disabled" {
                    disable-tunnel: [w386 _] -> w348
                    frame Disabled {
                      n119 = local read "Eye It Q"() -> (w387:refnum<queue>)
                      n120 = Dequeue Element(queue=w387) -> (element=w386:u32)  [unwired: 2 in, 3 out]
                    }
                    frame Enabled {
                    }
                  }
                  n121 = Flush Queue(queue=w355) -> (remaining elements=w354:dbl[])  [unwired: 1 in, 2 out]
                  n122 = Array Max & Min(array=w354) -> (max value=w353:dbl)  [unwired: 3 out]
                  n123 = To Unsigned Long Integer(number=w353) -> (unsigned 32bit integer=w351:u32)
                  n124 = Build Array(w351, w352, w348) -> (w350:u32[])
                  n125 = local read "PCO ref out"() -> (w357:refnum<file>)
                  n126 = local read "File Open"() -> (w356:bool)
                  n127 = Select(t=w380, s=w361, f=w373) -> (s? t:f=w367:i16)
                  n128 = Not(x=w361) -> (.not. x?=w360:bool)
                  n129 = call <vilib>:"GetImageBuffer.vi"("ph"=w379, "BuffIn"=w364, "BuffNr"=w367, "error in (no error)"=w378, "xRes"=w368, "yRes"=w370, "Bitresolution"=w369) -> ("hout"=w366:u64, "BuffOut"=w363:u16[], "error out"=w365:errorcluster)  [unwired: 5 in, 1 out]
                  n130 = local read "PCO Recording"() -> (w385:bool)
                  n131 = Unbundle By Name(w378) -> ("status"=w376:bool)
                  n132 = local write "bUseBuffer0"(w361) -> ()
                  n133 = local write "bUseBuffer1"(w360) -> ()
                  n134 = Not(x=w385) -> (.not. x?=w377:bool)
                  n135 = Or(x=w377, y=w376) -> (x .or. y?=w375:bool)
                  n136 = Reshape Array(w363, w370, w368) -> (w349:u16[][])
                  n137 = call "PCO File Save.vi"("Red, PCO/ Eye Iterations, Time"=w350, "Eye Track Info"=w347, "Ignore PCO"="Ignore PCO", "PCO Array"=w349, "File Open"=w356, "PCO Ref In"=w357) -> ("PCO Ref Out"=→"PCO Ref Out 2":refnum<file>)  [unwired: 3 in]
                  n138 = case shown="False" w356 {
                    tunnel: w349 -> [w397 _]
                    frame False {
                      "PCO Image" <- w397
                    }
                    frame True {
                    }
                  }
                }
                n139 = call <vilib>:"CancelImages.vi"("error in (no error)"=w308, "ph"=w309) -> ("error out"=w312:errorcluster, "hout"=w311:u64)  [unwired: 1 in, 1 out]
                n140 = call <vilib>:"SetRecordingState.vi"("ErrorIn"=w312, "RecordingState"=w343, "ph"=w311) -> ("ErrorOut"=w341:errorcluster, "hout"=w342:u64)  [unwired: 2 in, 1 out]
                n141 = while {
                  tunnel: [w436] -> w307
                  tunnel: w341 -> [w437]
                  tunnel: w342 -> [w438]
                  tunnel: [w433] -> _
                  stop <- w434 continue-if-true
                  # "Verify that recording is stopped before proceeding"
                  n142 = call <vilib>:"GetRecordingState.vi"("ErrorIn"=w437, "ph"=w438) -> ("ErrorOut"=w436:errorcluster, "RecordingState"=w435:u16, "hout"=w433:u64)  [unwired: 2 in, 1 out]
                  n143 = Not Equal To 0?(x=w435) -> (x != 0?=w434:bool)
                }
                n144 = call <vilib>:"Simple Error Handler.vi"("error in (no error)"=w307) -> ()  [unwired: 4 in, 5 out]
              }
              frame #1 {
                n145 = local write "PCO Recording"(FALSE ("Record")) -> ()
              }
            }
          }
        }
        n146 = Wait (ms) "Loop Wait"(milliseconds to wait=w248) -> ()  [unwired: 1 out]
        "PCO Recording" <- w236
      }
    }
    frame #2 {
      # "Free up any allocated buffers and close the camera communication channel"
      # "Quit:"
      n147 = call <vilib>:"Cleanup.vi"("error in (no error)"=w455, "ph"=w456) -> ("error out"=w457:errorcluster, "hout"=w458:u64)  [unwired: 8 in]
      n148 = call <vilib>:"CloseCamera.vi"("ErrorIn"=w457, "Handle in"=w458) -> ("ErrorOut"=w460:errorcluster)  [unwired: 1 in, 2 out]
      n149 = call <vilib>:"Simple Error Handler.vi"("error in (no error)"=w460) -> ()  [unwired: 4 in, 5 out]
      n150 = local write "bClose"(TRUE) -> ()
    }
  }
  n151 = local write "Relative \nRand Dist"(sgl 0.0 ("Rand Dist")) -> ()
  n152 = local write "Lick Begin \n- RZ One"(w1) -> ()
  n153 = local write "Small Stim"(w1) -> ()
  n154 = local write "Stim\nReceived"(w1) -> ()
  n155 = local write "False Alarm"(w1) -> ()
  n156 = case shown="True" "Test Encoder" {
    tunnel: [i64 20 ("Test Encoder Speed \n(Timed Loop Period)") "Test Encoder Speed \n(Timed Loop Period)"] -> w13
    frame False {
    }
    frame True {
    }
  }
  n157 = local write "UDP test"(0 ("Stim Identity")) -> ()
  n158 = call <vilib>:"DAQmx Create Task.vi"("new task name"="WheelEncoder", "global virtual channels"=w80) -> ("task out"=w53:refnum<k21>, "error out"=w52:errorcluster)  [unwired: 12 in]
  n159 = call <vilib>:"DAQmx Start Task.vi"("task/channels in"=w53, "error in"=w52) -> ("task out"=w83:refnum<k21>, "error out"=w82:errorcluster)  [unwired: 12 in]
  n160 = node-c288(w13) -> (w27:T6)  [unwired: 3 in]
  n161 = call <vilib>:"DAQmx Configure Input Buffer.vi"("task/channels in"=refnum<k21> "LickDetection", "buffer size (in samples per channel)"=u32 2500000) -> ("task out"=w46:refnum<k21>, "error out"=w44:errorcluster)  [unwired: 12 in]
  n162 = call <vilib>:"DAQmx Start Task.vi"("task/channels in"=w46, "error in"=w44) -> ("task out"=w48:refnum<k21>, "error out"=w47:errorcluster)  [unwired: 12 in]
  n163 = call "Simulate Signal2"("Offset"=2.5, "Frequency"=20.0, "Amplitude"=2.5, "Phase"=0.0) -> ("Square"=w93:dynamicdata, "error out"=w87:errorcluster)  [unwired: 10 in]
  n164 = call "Convert from Dynamic Data2"("Dynamic Data Type"=w93) -> ("Array"=w88:dbl[][])  [unwired: 3 in]
  n165 = call-poly <vilib>:"DAQmx Write.vi"("task/channels in"=refnum<k21> "Volt Trigger", "auto start"=FALSE, "data"=w88, "error in"=w87) -> ("task out"=w99:refnum<k21>, "error out"=w98:errorcluster)  [unwired: 9 in, 1 out]
  n166 = while {
    tunnel: w99 -> [w467]
    tunnel: [w465] -> w85
    tunnel: w98 -> [w466]
    tunnel: [w464] -> w84
    stop <- "Close Trigger 2" stop-if-true
    n167 = call <vilib>:"DAQmx Start Task.vi"("task/channels in"=w467, "error in"=w466) -> ("task out"=w465:refnum<k21>, "error out"=w464:errorcluster)  [unwired: 12 in]
  }
  n168 = call <vilib>:"DAQmx Stop Task.vi"("task/channels in"=w85, "error in"=w84) -> ("task out"=w95:refnum<k21>, "error out"=w94:errorcluster)  [unwired: 12 in]
  n169 = call <vilib>:"DAQmx Clear Task.vi"("task in"=w95, "error in"=w94) -> ("error out"=w100:errorcluster)  [unwired: 13 in]
  n170 = call <vilib>:"Simple Error Handler.vi"("type of dialog (OK msg:1)"=w97, "error in (no error)"=w100) -> ()  [unwired: 3 in, 5 out]
  n171 = Obtain Queue(max queue size (-1, unlimited)=1, name (unnamed)="Timer" ("format string"), element data type=0.0 ("Elapsed Time")) -> (queue out=w36:refnum<queue>, error out=w35:errorcluster)  [unwired: 2 in, 1 out]
  n172 = while {
    stop <- w468 stop-if-true
    n173 = event shown="[2] Timeout" {
      selector: _ -> [w470 w475 w477]
      dyn-events: [w470 w475 w477] -> _
      timeout: 1000 -> [_ _ _]
      tunnel: [_ _ w476] -> w468
      event Application Instance Close? {
        n174 = event-data() -> ()  [unwired: 1 in, 1 out]
        n175 = event-data("SilentShutdown"=FALSE, "Discard?"=TRUE) -> ()  [unwired: 1 in, 1 out]
      }
      event Panel Close? {
        n176 = event-data() -> ()  [unwired: 1 in, 1 out]
        n177 = One Button Dialog(message="Please click on 'Stop'\nbutton before closing!") -> (true=w473:bool)  [unwired: 1 in]
        n178 = event-data("Discard?"=w473) -> ()  [unwired: 1 in, 1 out]
      }
      event Timeout {
        n179 = event-data() -> ()  [unwired: 1 in, 3 out]
        n180 = local read "bClose"() -> (w476:bool)
      }
    }
  }
  n181 = String To IP(1:"169.230.68.195" ("name")) -> ()  [unwired: 1 out]
  n182 = UDP Open(11:u16 8888 ("Local Port")) -> (port=w31:refnum<k16>, 0:w30:errorcluster)  [unwired: 1 in, 4 out]
  n183 = timed-loop {
    tunnel: w83 -> [w625]
    tunnel: w82 -> [w616]
    shift-right: [w536] -> _
    shift-left: _ -> [w588]
    tunnel: w48 -> [w606]
    tunnel: w47 -> [w605]
    tunnel: refnum<k21> "LickValve" ("task/channels in") -> [w595]
    tunnel: [w594] -> w40
    tunnel: [w593] -> w39
    shift-right: [w589] -> _
    shift-left: _ -> [w570]
    tunnel: w36 -> [w585]
    tunnel: w35 -> [w584]
    tunnel: w31 -> [w574]
    tunnel: w30 -> [w573]
    tunnel: [w572] -> w29
    tunnel: [w571] -> w28
    timing: w27 -> [_]
    timing-out: [_] -> w26
    tunnel: w17 -> [w566]
    tunnel: w16 -> [w565]
    shift-right: [w550] -> _
    shift-left: 0.0 -> [w549]
    shift-right: [w540] -> _
    shift-left: _ -> [w539]
    tunnel: w8 -> [w531]
    tunnel: w7 -> [w530]
    tunnel: w4 -> [w528]
    tunnel: w3 -> [w527]
    shift-right: [w487] -> _
    shift-left: _ -> [w486]
    i -> [w516]
    stop <- "Stop Encoder" stop-if-true
    # "Static or Moving Stim"
    # "Left or Right or No Cue"
    # "Left or Right Stim"
    # "Short or Long Stim"
    # "Stim, Lick?, Reward?, \nDist at Lick or Time of Lick"
    # "Total Dist traveled,\nRand Dist Generated"
    n184 = node-c288() -> ()  [unwired: 1 in, 1 out]
    n185 = local read "Test Encoder"() -> (w543:bool)
    n186 = Dequeue Element(queue=w531, error in (no error)=w530) -> (element=w529:string)  [unwired: 1 in, 3 out]
    n187 = Or(x=w543, y="NewTrial") -> (x .or. y?=w548:bool)
    n188 = Flush Queue(queue=w566, error in (no error)=w565) -> (remaining elements=w567:i32[])  [unwired: 2 out]
    n189 = case shown="\"N\"" w529 {
      tunnel: [FALSE TRUE FALSE] -> w500
      frame "N" {
      }
      frame "S" {
      }
      frame "O", Default {
      }
    }
    "Small Stim" <- w500
    n190 = case shown="True" "NewTrial" {
      frame False {
      }
      frame True {
        n191 = local write "Rand Number Created"(FALSE ("Rand Number Created")) -> ()
        n192 = local write "UDP test"(0 ("UDP test")) -> ()
      }
    }
    n193 = local read "Stim\nReceived"() -> (w504:bool)
    n194 = local read "Stim\nReceived"() -> (w498:bool)
    n195 = Array Max & Min(array=w567) -> (max value=w494:i32)  [unwired: 3 out]
    n196 = case shown="True" w548 {
      tunnel: w625 -> [w1152 w1158]
      tunnel: [w1152 w1155] -> w623
      tunnel: [w1151 w1154] -> w622
      tunnel: w616 -> [w1151 w1153]
      frame False {
      }
      frame True {
        n197 = call <vilib>:"DAQmx Stop Task.vi"("task/channels in"=w1158, "error in"=w1153) -> ("task out"=w1157:refnum<k21>, "error out"=w1156:errorcluster)  [unwired: 12 in]
        n198 = call <vilib>:"DAQmx Start Task.vi"("task/channels in"=w1157, "error in"=w1156) -> ("task out"=w1155:refnum<k21>, "error out"=w1154:errorcluster)  [unwired: 12 in]
      }
    }
    n199 = call-poly <vilib>:"DAQmx Read.vi"("task/channels in"=w606, "error in"=w605) -> ("data"=w603:digitalwaveform)  [unwired: 11 in, 2 out]
    n200 = Boolean To (0,1)(Boolean="NewTrial") -> (0, 1=w621:i16)
    n201 = Not Equal To 0?(x=w494) -> (x != 0?=w564:bool)
    n202 = Equal To 0?(x=w494) -> (x = 0?=w505:bool)
    n203 = Not(x=w504) -> (.not. x?=w503:bool)
    n204 = Not(x=w498) -> (.not. x?=w499:bool)
    n205 = Unbundle By Name(w603) -> ("Y"=w604:digitaldata)
    n206 = Greater?(x=w494, y=1) -> (0:w507:bool)
    n207 = Format Into String(format string="%d", w621) -> (resulting string=w563:string)  [unwired: 2 in, 1 out]
    n208 = case shown="True" w564 {
      tunnel: w494 -> [_ w716]
      frame False {
      }
      frame True {
        n209 = local write "Relative \nRand Dist"(0.0 ("Relative \nRand Dist")) -> ()
        "UDP test" <- w716
      }
    }
    n210 = Equal?(x=w494, y=1) -> (x = y?=w496:bool)
    n211 = And(x=w503, y=w507) -> (x .and. y?=w506:bool)
    n212 = case shown="True" w505 {
      frame False {
      }
      frame True {
        w630 = 0 ("Stim")
        n213 = local write "Stim\nReceived"(FALSE ("Stim\nReceived")) -> ()
        n214 = local write "Stim 2"(w630) -> ()
        n215 = local write "Stim"(w630) -> ()
      }
    }
    n216 = Unbundle By Name(w604) -> ("data"=w602:u8[][])
    n217 = And(x=w499, y=w496) -> (x .and. y?=w497:bool)
    n218 = case shown="True" w506 {
      frame False {
      }
      frame True {
        "Stim" <- 2 ("Stim")
      }
    }
    n219 = local read "Rand Number Created"() -> (w556:bool)
    n220 = case shown="True" w497 {
      frame False {
      }
      frame True {
        "Stim 2" <- 1 ("Stim")
      }
    }
    n221 = call-poly <vilib>:"DAQmx Read.vi"("task/channels in"=w623, "timeout"=-1.0, "error in"=w622) -> ("data"=w547:dbl)  [unwired: 10 in, 2 out]
    n222 = case shown="True" w543 {
      tunnel: [0.0 w669] -> w550
      tunnel: w549 -> [_ w670]
      tunnel: [w667 w669] -> w546
      tunnel: w547 -> [w667 _]
      tunnel: [w667 w669] -> w545
      frame False {
      }
      frame True {
        n223 = Add(x=w670, y=0.75) -> (x+y=w669:dbl)
      }
    }
    "Total Dist Travelled" <- w546
    n224 = Array Max & Min(array=w602) -> (max value=w540:u8)  [unwired: 3 out]
    n225 = local read "UDP test"() -> (w559:i32)
    n226 = Not Equal?(x=w539, y=w540) -> (x != y?=w538:bool)
    n227 = Equal To 0?(x=w559) -> (x = 0?=w558:bool)
    n228 = Not(x=w556) -> (.not. x?=w555:bool)
    n229 = Boolean To (0,1)(Boolean=w538) -> (0, 1=→"Lick Waveform":i16)
    n230 = And(x=w558, y=w555) -> (x .and. y?=w557:bool)
    n231 = Tick Count (ms)() -> (millisecond timer value=w569:u32)
    n232 = case shown="\"Cued Attention Task \"" "MODE" {
      tunnel: [w740 w780 w876 w1018 w1093] -> w536
      tunnel: w538 -> [w746 w776 w873 w1015 w1074]
      tunnel: [w746 w776 w873 w1015 w1074] -> w614
      tunnel: [u32 0 w779 w871 w1013 w1089] -> w611
      tunnel: w569 -> [w743 w772 w859 w1005 w1068]
      tunnel: w546 -> [w744 w782 w878 w1020 w1095]
      tunnel: w588 -> [w741 w783 w864 w1010 w1096]
      tunnel: [w740 w781 w877 w1019 w1094] -> w607
      tunnel: "Give Soymilk" -> [w738 w781 w877 w1019 w1094]
      tunnel: "Droplet Duration" -> [w742 w786 w881 w1023 w1099]
      tunnel: "Lick Window(ms)" -> [_ _ w872 w1014 w1073]
      tunnel: [u32 0 ("millisecond timer value") w778 w875 w1017 w1092] -> w589
      tunnel: w570 -> [_ w787 w882 w1024 w1082]
      tunnel: "Reward Zone Start" -> [_ w784 w879 w1021 w1097]
      tunnel: "Reward Zone Finish" -> [_ w785 w880 w1022 w1098]
      tunnel: [0 0 0 0 w1070] -> w487
      tunnel: w486 -> [_ _ _ _ w1076]
      frame "Run Training" {
        (unwired) FALSE
        n233 = case shown="True" "Distance \nTriggered" {
          tunnel: [w748 w752] -> w740
          tunnel: w744 -> [_ w755]
          tunnel: w738 -> [w748 w749]
          tunnel: w743 -> [_ w754]
          tunnel: w742 -> [_ w753]
          tunnel: w741 -> [_ _]
          frame False {
          }
          frame True {
            n234 = Quotient & Remainder(x=w755, y="Reward\n Distance") -> (x-y*floor(x/y)=w757:dbl)  [unwired: 1 out]
            n235 = Subtract(x="Reward\n Distance", y=1.0) -> (x-y=w758:dbl)
            n236 = Greater?(x=w757, y=w758) -> (0:w750:bool)
            n237 = Or(x=w749, y=w750) -> (x .or. y?=w751:bool)
            n238 = case shown="True" w751 {
              tunnel: [FALSE w762] -> w752
              tunnel: w754 -> [_ w765]
              tunnel: w753 -> [_ w761]
              frame False {
              }
              frame True {
                n239 = local read "Reward Start (ms) - \nRun Train"() -> (w766:u32)
                n240 = Subtract(x=w765, y=w766) -> (x-y=w764:u32)
                n241 = Greater?(x=w764, y=w761) -> (0:w763:bool)
                n242 = case shown="False" w763 {
                  tunnel: [TRUE FALSE] -> w762
                  frame False {
                  }
                  frame True {
                  }
                }
              }
            }
            n243 = case shown="True" w750 {
              tunnel: w754 -> [_ w769]
              frame False {
              }
              frame True {
                "Reward Start (ms) - \nRun Train" <- w769
              }
            }
          }
        }
      }
      frame "Discrimination Only Task" {
        (unwired) FALSE
        n244 = local read "Stim"() -> (w771:i32)
        n245 = Not Equal To 0?(x=w787) -> (x != 0?=w791:bool)
        n246 = To Single Precision Float(number=w782) -> (single precision float=w793:sgl)
        n247 = To Single Precision Float(number=w782) -> (single precision float=w792:sgl)
        n248 = Greater?(x=w771, y=1) -> (0:w774:bool)
        n249 = Or(x=w791, y=w774) -> (x .or. y?=w773:bool)
        n250 = case shown="True" w773 {
          tunnel: [w806 w824] -> w777
          tunnel: [sgl 0.0 w813] -> w779
          tunnel: w793 -> [_ w815]
          tunnel: w784 -> [_ w821]
          tunnel: w772 -> [_ _]
          tunnel: w785 -> [_ w811]
          tunnel: w776 -> [_ w830]
          tunnel: w776 -> [_ _]
          tunnel: [0 1] -> w790
          tunnel: [w806 w817] -> w788
          frame False {
            w806 = FALSE
          }
          frame True {
            n251 = local read "Stim Start Dist\n(Discrim Only)"() -> (w816:sgl)
            n252 = Increment(x=w811) -> (x+1=w812:sgl)
            n253 = Add(x=sgl 5.0, y=w811) -> (x+y=w810:sgl)
            n254 = Subtract(x=w815, y=w816) -> (x-y=w813:sgl)
            n255 = In Range and Coerce(upper limit=w812, x=w813, lower limit=w811) -> (In Range?=w814:bool)  [unwired: 1 out]
            n256 = Greater?(x=w813, y=w810) -> (0:w818:bool)
            n257 = In Range and Coerce(upper limit=w811, x=w813, lower limit=w821) -> (In Range?=w829:bool)  [unwired: 1 out]
            n258 = And(x=w829, y=w830) -> (x .and. y?=w828:bool)
            n259 = flat-sequence {
              tunnel: w828 -> [w835]
              tunnel: [w836] -> w827
              tunnel: w814 -> [w833]
              tunnel: [w833] -> w826
              tunnel: w827 -> [w841]
              tunnel: w826 -> [w839]
              tunnel: [w841] -> w820
              tunnel: [w840] -> w819
              tunnel: [w849] -> w823
              tunnel: [w850] -> w825
              tunnel: w820 -> [w850]
              tunnel: w819 -> [w849]
              tunnel: w818 -> [w848]
              tunnel: [w847] -> w817
              frame #0 {
                n260 = local read "Lick Begin \n- RZ One"() -> (w831:bool)
                n261 = Not(x=w831) -> (.not. x?=w832:bool)
                n262 = And(x=w832, y=w835) -> (x .and. y?=w834:bool)
                n263 = case shown="True" w834 {
                  selector: w834 -> [w837 w838]
                  tunnel: [w837 w838] -> w836
                  frame False {
                  }
                  frame True {
                    "Lick Begin \n- RZ One" <- w838
                  }
                }
              }
              frame #1 {
                n264 = case shown="True" w839 {
                  tunnel: [FALSE w843] -> w840
                  frame False {
                  }
                  frame True {
                    n265 = local read "Lick Begin \n- RZ One"() -> (w844:bool)
                    n266 = case shown="False" w844 {
                      tunnel: [w845 FALSE] -> w843
                      frame False {
                        w845 = TRUE
                        n267 = local write "Lick Begin \n- RZ One"(w845) -> ()
                      }
                      frame True {
                      }
                    }
                  }
                }
              }
              frame #2 {
                n268 = case shown="True" w848 {
                  selector: w848 -> [w851 w853]
                  tunnel: [w851 w853] -> w847
                  frame False {
                  }
                  frame True {
                    n269 = local write "Lick Begin \n- RZ One"(FALSE) -> ()
                  }
                }
              }
            }
            n270 = Or(x=w823, y=w825) -> (x .or. y?=w824:bool)
          }
        }
        n271 = case shown="True" w774 {
          tunnel: w792 -> [_ w856]
          tunnel: w772 -> [_ w855]
          frame False {
            n272 = local write "UDP test"(0 ("UDP test")) -> ()
          }
          frame True {
            "Stim Start Dist\n(Discrim Only)" <- w856
            "Stim Start Time\n(Discrim Only)" <- w855
          }
        }
        n273 = case shown="True" w783 {
          tunnel: [FALSE w798] -> w789
          tunnel: w786 -> [_ w800]
          tunnel: w772 -> [_ w799]
          frame False {
          }
          frame True {
            n274 = local read "Reward Start (ms) \n(Discrim Only)"() -> (w803:u32)
            n275 = Subtract(x=w799, y=w803) -> (x-y=w802:u32)
            n276 = Greater?(x=w802, y=w800) -> (0:w801:bool)
            n277 = case shown="True" w801 {
              tunnel: [TRUE FALSE] -> w798
              frame False {
              }
              frame True {
              }
            }
          }
        }
        n278 = case shown="False" w788 {
          tunnel: [w795 0] -> w778
          tunnel: w790 -> [w795 _]
          frame False {
          }
          frame True {
          }
        }
        n279 = case shown="True" w777 {
          tunnel: w772 -> [_ w794]
          frame False {
          }
          frame True {
            "Reward Start (ms) \n(Discrim Only)" <- w794
          }
        }
        n280 = Or(x=w777, y=w789) -> (x .or. y?=w780:bool)
      }
      frame "Discrimination Variant Task" {
        n281 = local read "Stim Variation"() -> (w870:i16)
        n282 = case shown="2" w870 {
          tunnel: [FALSE TRUE FALSE w905] -> w867
          frame 3, Default {
          }
          frame 4 {
          }
          frame 1 {
          }
          frame 2 {
            w905 = FALSE
            n283 = local write "Vert\nVariant"(w905) -> ()
          }
        }
        n284 = local read "Small Stim"() -> (w866:bool)
        n285 = flat-sequence {
          tunnel: w878 -> [w892]
          tunnel: [w893] -> w862
          tunnel: [w889] -> w861
          tunnel: w862 -> [w895]
          tunnel: w861 -> [w896]
          tunnel: [w896] -> w860
          tunnel: w859 -> [w894]
          frame #0 {
            n286 = local read "Stim"() -> (w890:i32)
            n287 = Greater?(x=w890, y=1) -> (0:w889:bool)
            n288 = To Single Precision Float(number=w892) -> (single precision float=w893:sgl)
          }
          frame #1 {
            n289 = case shown="True" w896 {
              selector: w896 -> [_ w899]
              tunnel: w895 -> [_ w901]
              tunnel: w894 -> [_ w900]
              frame False {
                n290 = local write "UDP test"(0 ("UDP test")) -> ()
              }
              frame True {
                n291 = local write "Stim"(1 ("Stim")) -> ()
                "Stim Start Dist \n(Discrim Vary)" <- w901
                "Stim Start Time\n(Discrim Vary)" <- w900
                "Stim\nReceived" <- w899
              }
            }
          }
        }
        n292 = And(x=w867, y=w866) -> (x .and. y?=w868:bool)
        n293 = flat-sequence {
          tunnel: w868 -> [w886]
          tunnel: [w888] -> w858
          frame #0 {
            n294 = case shown="True" w886 {
              frame False {
              }
              frame True {
                "Vert\nVariant" <- TRUE
              }
            }
          }
          frame #1 {
            n295 = local read "Vert\nVariant"() -> (w888:bool)
          }
        }
        n296 = To Single Precision Float(number=w878) -> (single precision float=w885:sgl)
        n297 = Not Equal To 0?(x=w882) -> (x != 0?=w884:bool)
        n298 = Or(x=w884, y=w860) -> (x .or. y?=w869:bool)
        n299 = case shown="True" w869 {
          selector: w869 -> [_ w911]
          tunnel: w885 -> [_ w921]
          tunnel: [0 w920] -> w883
          tunnel: [FALSE w919] -> w863
          tunnel: w880 -> [_ w918]
          tunnel: w879 -> [_ w917]
          tunnel: [FALSE w916] -> w874
          tunnel: w873 -> [_ w912]
          tunnel: w872 -> [_ w915]
          tunnel: w859 -> [_ w914]
          tunnel: [sgl 0.0 w913] -> w871
          tunnel: w858 -> [_ w910]
          frame False {
            (unwired) FALSE
          }
          frame True {
            n300 = case shown="True" w910 {
              tunnel: [w937 w968] -> w916
              tunnel: w921 -> [w928 _]
              tunnel: w917 -> [w934 _]
              tunnel: w918 -> [w925 _]
              tunnel: w912 -> [w943 w967]
              tunnel: [1 w973] -> w920
              tunnel: [w930 w969] -> w919
              tunnel: w911 -> [_ w976]
              tunnel: w915 -> [_ w975]
              tunnel: w914 -> [_ w974]
              tunnel: [w922 w972] -> w913
              frame False {
                (unwired) FALSE
                n301 = local read "Stim Start Dist \n(Discrim Vary)"() -> (w929:sgl)
                n302 = Increment(x=w925) -> (x+1=w926:sgl)
                n303 = Add(x=sgl 5.0, y=w925) -> (x+y=w924:sgl)
                n304 = Subtract(x=w928, y=w929) -> (x-y=w922:sgl)
                n305 = In Range and Coerce(upper limit=w926, x=w922, lower limit=w925) -> (In Range?=w927:bool)  [unwired: 1 out]
                n306 = Greater?(x=w922, y=w924) -> (0:w931:bool)
                n307 = In Range and Coerce(upper limit=w925, x=w922, lower limit=w934) -> (In Range?=w942:bool)  [unwired: 1 out]
                n308 = And(x=w942, y=w943) -> (x .and. y?=w941:bool)
                n309 = flat-sequence {
                  tunnel: w941 -> [w948]
                  tunnel: [w949] -> w940
                  tunnel: w927 -> [w946]
                  tunnel: [w946] -> w939
                  tunnel: w940 -> [w954]
                  tunnel: w939 -> [w952]
                  tunnel: [w954] -> w933
                  tunnel: [w953] -> w932
                  tunnel: [w962] -> w936
                  tunnel: [w963] -> w938
                  tunnel: w933 -> [w963]
                  tunnel: w932 -> [w962]
                  tunnel: w931 -> [w961]
                  tunnel: [w960] -> w930
                  frame #0 {
                    n310 = local read "Lick Begin \n- RZ One  2"() -> (w944:bool)
                    n311 = Not(x=w944) -> (.not. x?=w945:bool)
                    n312 = And(x=w945, y=w948) -> (x .and. y?=w947:bool)
                    n313 = case shown="True" w947 {
                      selector: w947 -> [w950 w951]
                      tunnel: [w950 w951] -> w949
                      frame False {
                      }
                      frame True {
                        "Lick Begin \n- RZ One  2" <- w951
                      }
                    }
                  }
                  frame #1 {
                    n314 = case shown="True" w952 {
                      tunnel: [FALSE w956] -> w953
                      frame False {
                      }
                      frame True {
                        n315 = local read "Lick Begin \n- RZ One  2"() -> (w957:bool)
                        n316 = case shown="False" w957 {
                          tunnel: [w958 FALSE] -> w956
                          frame False {
                            w958 = TRUE
                            n317 = local write "Lick Begin \n- RZ One  2"(w958) -> ()
                          }
                          frame True {
                          }
                        }
                      }
                    }
                  }
                  frame #2 {
                    n318 = case shown="True" w961 {
                      selector: w961 -> [w964 w966]
                      tunnel: [w964 w966] -> w960
                      frame False {
                      }
                      frame True {
                        n319 = local write "Lick Begin \n- RZ One  2"(FALSE) -> ()
                      }
                    }
                  }
                }
                n320 = Or(x=w936, y=w938) -> (x .or. y?=w937:bool)
              }
              frame True {
                n321 = case shown="True" w976 {
                  tunnel: w974 -> [_ w991]
                  tunnel: [FALSE w983] -> w968
                  tunnel: w975 -> [_ w986]
                  tunnel: [0 1] -> w973
                  tunnel: [u32 0 w988] -> w972
                  tunnel: [FALSE w985] -> w971
                  tunnel: [FALSE TRUE] -> _
                  tunnel: w967 -> [_ w982]
                  frame False {
                    (unwired) u32 0
                    (unwired) u32 0 ("Lick Window(ms) -\nEither Stim")
                  }
                  frame True {
                    n322 = local read "Stim Start Time\n(Discrim Vary)"() -> (w989:u32)
                    n323 = Subtract(x=w991, y=w989) -> (x-y=w987:u32)
                    n324 = To Single Precision Float(number=w987) -> (single precision float=w988:sgl)
                    n325 = Greater?(x=w986, y=w987) -> (0:w985:bool)
                    n326 = And(x=w982, y=w985) -> (x .and. y?=w983:bool)
                  }
                }
                n327 = Not(x=w971) -> (.not. x?=w970:bool)
                n328 = Or(x=w968, y=w970) -> (x .or. y?=w969:bool)
              }
            }
          }
        }
        n329 = case shown="True" w864 {
          tunnel: [FALSE w996] -> w865
          tunnel: w881 -> [_ w998]
          tunnel: w859 -> [_ w997]
          frame False {
          }
          frame True {
            n330 = local read "Reward Start (ms) \n(Discrim Vary)"() -> (w1001:u32)
            n331 = Subtract(x=w997, y=w1001) -> (x-y=w1000:u32)
            n332 = Greater?(x=w1000, y=w998) -> (0:w999:bool)
            n333 = case shown="True" w999 {
              tunnel: [TRUE FALSE] -> w996
              frame False {
              }
              frame True {
              }
            }
          }
        }
        n334 = case shown="True" w863 {
          tunnel: [w993 0] -> w875
          tunnel: w883 -> [w993 _]
          frame False {
            (unwired) TRUE
          }
          frame True {
          }
        }
        n335 = case shown="True" w874 {
          tunnel: w859 -> [_ w992]
          frame False {
          }
          frame True {
            "Reward Start (ms) \n(Discrim Vary)" <- w992
          }
        }
        n336 = Or(x=w874, y=w865) -> (x .or. y?=w876:bool)
      }
      frame "Alternating Variant Presentation" {
        n337 = flat-sequence {
          tunnel: w1020 -> [w1031]
          tunnel: [w1032] -> w1008
          tunnel: [w1028] -> w1007
          tunnel: w1008 -> [w1034]
          tunnel: w1007 -> [w1035]
          tunnel: [w1035] -> w1006
          tunnel: w1005 -> [w1033]
          frame #0 {
            n338 = local read "Stim"() -> (w1029:i32)
            n339 = Greater?(x=w1029, y=1) -> (0:w1028:bool)
            n340 = To Single Precision Float(number=w1031) -> (single precision float=w1032:sgl)
          }
          frame #1 {
            n341 = case shown="True" w1035 {
              selector: w1035 -> [_ w1038]
              tunnel: w1034 -> [_ w1040]
              tunnel: w1033 -> [_ w1039]
              frame False {
                n342 = local write "UDP test"(0 ("UDP test")) -> ()
              }
              frame True {
                n343 = local write "Stim"(1 ("Stim")) -> ()
                "Stim Start Dist \n(Discrim Vary) 2" <- w1040
                "Stim Start Time\n(Discrim Vary)  2" <- w1039
                "Stim\nReceived 2" <- w1038
              }
            }
          }
        }
        n344 = To Single Precision Float(number=w1020) -> (single precision float=w1027:sgl)
        n345 = Not Equal To 0?(x=w1024) -> (x != 0?=w1026:bool)
        n346 = Or(x=w1026, y=w1006) -> (x .or. y?=w1012:bool)
        n347 = case shown="True" w1012 {
          tunnel: w1027 -> [_ _]
          tunnel: [0 1] -> w1025
          tunnel: [FALSE w1054] -> w1009
          tunnel: w1022 -> [_ _]
          tunnel: w1021 -> [_ _]
          tunnel: [FALSE w1053] -> w1016
          tunnel: w1015 -> [_ w1049]
          tunnel: w1014 -> [_ w1052]
          tunnel: w1005 -> [_ w1051]
          tunnel: [sgl 0.0 w1050] -> w1013
          frame False {
            (unwired) FALSE
          }
          frame True {
            n348 = local read "Stim Start Time\n(Discrim Vary)  2"() -> (w1046:u32)
            n349 = Subtract(x=w1051, y=w1046) -> (x-y=w1045:u32)
            n350 = To Single Precision Float(number=w1045) -> (single precision float=w1050:sgl)
            n351 = Greater?(x=w1052, y=w1045) -> (0:w1048:bool)
            n352 = And(x=w1049, y=w1048) -> (x .and. y?=w1053:bool)
            n353 = Not(x=w1048) -> (.not. x?=w1047:bool)
            n354 = Or(x=w1053, y=w1047) -> (x .or. y?=w1054:bool)
          }
        }
        n355 = case shown="True" w1010 {
          tunnel: [FALSE w1060] -> w1011
          tunnel: w1023 -> [_ w1062]
          tunnel: w1005 -> [_ w1061]
          frame False {
          }
          frame True {
            n356 = local read "Reward Start (ms) \n(Discrim Vary) 2"() -> (w1065:u32)
            n357 = Subtract(x=w1061, y=w1065) -> (x-y=w1064:u32)
            n358 = Greater?(x=w1064, y=w1062) -> (0:w1063:bool)
            n359 = case shown="True" w1063 {
              tunnel: [TRUE FALSE] -> w1060
              frame False {
              }
              frame True {
              }
            }
          }
        }
        n360 = case shown="True" w1009 {
          tunnel: [w1057 0] -> w1017
          tunnel: w1025 -> [w1057 _]
          frame False {
            (unwired) TRUE
          }
          frame True {
          }
        }
        n361 = case shown="True" w1016 {
          tunnel: w1005 -> [_ w1056]
          frame False {
          }
          frame True {
            "Reward Start (ms) \n(Discrim Vary) 2" <- w1056
          }
        }
        n362 = Or(x=w1016, y=w1011) -> (x .or. y?=w1018:bool)
      }
      frame "Cued Attention Task " {
        (unwired) FALSE
        n363 = local read "Stim"() -> (w1080:i32)
        n364 = Not Equal To 0?(x=w1082) -> (x != 0?=w1081:bool)
        n365 = local read "Stim 2"() -> (w1072:i32)
        n366 = Equal?(x=1, y=w1072) -> (x = y?=w1078:bool)
        n367 = To Single Precision Float(number=w1095) -> (single precision float=w1104:sgl)
        n368 = To Single Precision Float(number=w1095) -> (single precision float=w1103:sgl)
        n369 = Greater?(x=w1080, y=1) -> (0:w1090:bool)
        n370 = Or(x=w1081, y=w1090) -> (x .or. y?=w1088:bool)
        n371 = case shown="True" w1078 {
          tunnel: w1068 -> [_ w1109]
          frame False {
            n372 = local write "UDP test"(0 ("UDP test")) -> ()
          }
          frame True {
            "Diag Start Time" <- w1109
          }
        }
        n373 = Not Equal To 0?(x=w1076) -> (x != 0?=w1075:bool)
        n374 = Or(x=w1075, y=w1078) -> (x .or. y?=w1077:bool)
        n375 = case shown="True" w1088 {
          tunnel: [w1121 FALSE] -> w1086
          tunnel: w1104 -> [_ _]
          tunnel: w1097 -> [_ _]
          tunnel: w1098 -> [_ _]
          tunnel: w1074 -> [w1125 _]
          tunnel: [1 0] -> w1102
          tunnel: [w1120 FALSE] -> w1100
          tunnel: w1073 -> [w1124 _]
          tunnel: w1068 -> [w1129 _]
          tunnel: [w1127 sgl 0.0] -> w1089
          frame True {
            n376 = local read "Stim Start Time\n(Cue Only)"() -> (w1126:u32)
            n377 = Subtract(x=w1129, y=w1126) -> (x-y=w1123:u32)
            n378 = To Single Precision Float(number=w1123) -> (single precision float=w1127:sgl)
            n379 = Greater?(x=w1124, y=w1123) -> (0:w1122:bool)
            n380 = And(x=w1125, y=w1122) -> (x .and. y?=w1121:bool)
            n381 = Not(x=w1122) -> (.not. x?=w1120:bool)
            n382 = case shown="True" w1120 {
              frame False {
              }
              frame True {
                n383 = local write "Licked"(FALSE ("Licked")) -> ()
              }
            }
            n384 = case shown="True" w1121 {
              selector: w1121 -> [_ w1131]
              frame False {
              }
              frame True {
                "Licked" <- w1131
              }
            }
          }
          frame False {
          }
        }
        n385 = case shown="True" w1090 {
          tunnel: w1103 -> [_ w1150]
          tunnel: w1068 -> [_ w1149]
          frame False {
            n386 = local write "UDP test"(0 ("UDP test")) -> ()
          }
          frame True {
            "Stim Start Dist \n(Cue Only)" <- w1150
            "Stim Start Time\n(Cue Only)" <- w1149
          }
        }
        n387 = case shown="True" w1077 {
          tunnel: w1074 -> [_ _]
          tunnel: w1073 -> [_ w1116]
          tunnel: w1068 -> [_ w1115]
          tunnel: [FALSE w1114] -> w1071
          tunnel: [0 1] -> w1069
          frame False {
          }
          frame True {
            n388 = local read "Diag Start Time"() -> (w1119:u32)
            n389 = Subtract(x=w1115, y=w1119) -> (x-y=w1118:u32)
            n390 = Greater?(x=w1116, y=w1118) -> (0:w1114:bool)
            n391 = And(x=w1114, y=TRUE) -> (x .and. y?=→"False Alarm":bool)
          }
        }
        n392 = case shown="True" w1096 {
          tunnel: [FALSE w1140] -> w1101
          tunnel: w1099 -> [_ w1142]
          tunnel: w1068 -> [_ w1141]
          frame False {
          }
          frame True {
            n393 = local read "Reward Start (ms) \n(Cue Only)"() -> (w1145:u32)
            n394 = Subtract(x=w1141, y=w1145) -> (x-y=w1144:u32)
            n395 = Greater?(x=w1144, y=w1142) -> (0:w1143:bool)
            n396 = case shown="True" w1143 {
              tunnel: [TRUE FALSE] -> w1140
              frame False {
              }
              frame True {
              }
            }
          }
        }
        n397 = case shown="False" w1071 {
          tunnel: [0 w1107] -> w1070
          tunnel: w1069 -> [_ w1107]
          frame False {
            n398 = local write "False Alarm"(FALSE ("False Alarm")) -> ()
          }
          frame True {
          }
        }
        n399 = local read "Licked"() -> (w1087:bool)
        n400 = Not(x=w1087) -> (.not. x?=w1083:bool)
        n401 = And(x=w1083, y=w1086) -> (x .and. y?=w1085:bool)
        n402 = Or(x=w1083, y=w1100) -> (x .or. y?=w1084:bool)
        n403 = case shown="True" w1084 {
          tunnel: [w1137 0] -> w1092
          tunnel: w1102 -> [w1137 _]
          frame False {
          }
          frame True {
          }
        }
        n404 = case shown="True" w1085 {
          tunnel: w1068 -> [_ w1136]
          frame False {
          }
          frame True {
            "Reward Start (ms) \n(Cue Only)" <- w1136
          }
        }
        n405 = Or(x=w1085, y=w1101) -> (x .or. y?=w1093:bool)
      }
    }
    n406 = case shown="True" w557 {
      tunnel: "Rand Stim\nDist Interval" -> [_ w708]
      tunnel: ["O" w707] -> w553
      tunnel: [0.0 w696] -> w552
      tunnel: ["O" w693] -> w535
      tunnel: [i16 0 w689] -> w534
      frame False {
      }
      frame True {
        # "Rand Stim Version"
        # "Rand Stim"
        # "Random Distance"
        n407 = Random Number (0-1)() -> (number: 0 to 1=w702:dbl)
        n408 = Random Number (0-1)() -> (number: 0 to 1=w698:dbl)
        n409 = Random Number (0-1)() -> (number: 0 to 1=w695:dbl)
        n410 = Quotient & Remainder(x=w702, y=0.3) -> (x-y*floor(x/y)=w705:dbl)  [unwired: 1 out]
        n411 = Greater Or Equal?(x=w698, y=0.5 ("x")) -> (x >= y?=w697:bool)
        n412 = Greater Or Equal?(x=w695, y=0.5 ("x")) -> (x >= y?=w691:bool)
        n413 = Boolean To (0,1)(Boolean=w697) -> (0, 1=w692:i16)
        n414 = Add(x=0.1 ("y"), y=w705) -> (x+y=w704:dbl)
        n415 = case shown="True" w691 {
          tunnel: [i16 1 i16 3] -> w690
          frame False {
          }
          frame True {
          }
        }
        n416 = Multiply(x=100.0, y=w704) -> (x*y=w700:dbl)
        n417 = Add(x=w708, y=w700) -> (x+y=w696:dbl)
        n418 = Add(x=w692, y=w690) -> (x+y=w689:i16)
        n419 = case shown="0, Default" w692 {
          tunnel: ["D" "V"] -> w707
          frame 0, Default {
          }
          frame 1 {
          }
        }
        n420 = case shown="1, Default" w690 {
          tunnel: ["Baseline" "Variant"] -> w693
          frame 1, Default {
          }
          frame 3 {
          }
        }
      }
    }
    n421 = flat-sequence {
      tunnel: w552 -> [w675]
      tunnel: w553 -> [w674]
      tunnel: w535 -> [w673]
      tunnel: w534 -> [w672]
      tunnel: [w683] -> w554
      tunnel: [w682] -> w501
      tunnel: [w681] -> w502
      frame #0 {
        n422 = Not Equal To 0?(x=w675) -> (x != 0?=w676:bool)
        n423 = case shown="True" w676 {
          tunnel: w675 -> [_ w680]
          tunnel: w674 -> [_ w679]
          tunnel: w673 -> [_ w678]
          tunnel: w672 -> [_ w677]
          frame False {
          }
          frame True {
            "Relative \nRand Dist" <- w680
            "Stim Identity" <- w679
            "Varied Stim" <- w678
            "Stim Variation" <- w677
          }
        }
      }
      frame #1 {
        n424 = local read "Relative \nRand Dist"() -> (w683:dbl)
        n425 = local read "Stim Variation"() -> (w681:i16)
        n426 = local read "Stim Identity"() -> (w682:string)
        n427 = Not Equal To 0?(x=w683) -> (x != 0?=→"Rand Number Created":bool)
      }
    }
    n428 = Build Array(w547, w552) -> (w615:dbl[])
    n429 = To Single Precision Float(number=w615) -> (single precision float=w551:sgl[])
    n430 = To Single Precision Float(number=w545) -> (single precision float=w619:sgl)
    n431 = Format Into String(format string="%f", w619) -> (resulting string=w490:string)  [unwired: 2 in, 1 out]
    n432 = Dequeue Element(queue=w528, error in (no error)=w527) -> (element=w482:string)  [unwired: 1 in, 3 out]
    n433 = String Subset(string=w482, length (rest)=1 ("length (rest)")) -> (substring=w523:string)  [unwired: 1 in]
    n434 = String Subset(string=w482, offset (0)=2, length (rest)=1 ("length (rest)")) -> (substring=w522:string)
    n435 = String Subset(string=w482, offset (0)=1, length (rest)=1 ("length (rest)")) -> (substring=w521:string)
    n436 = String Subset(string=w482, offset (0)=3, length (rest)=1 ("length (rest)")) -> (substring=w483:string)
    n437 = String Subset(string=w482, offset (0)=4, length (rest)=1 ("length (rest)")) -> (substring=w481:string)
    n438 = case shown="\"R\"" w522 {
      tunnel: [0 1 0 2] -> w519
      frame "O", Default {
      }
      frame "R" {
      }
      frame "X" {
      }
      frame "L" {
      }
    }
    n439 = case shown="\"2\"" w481 {
      tunnel: [0 1 2] -> w479
      frame "O", Default {
      }
      frame "1" {
      }
      frame "2" {
      }
    }
    n440 = case shown="\"S\"" w523 {
      tunnel: [0 1 2] -> w511
      frame "O", Default {
      }
      frame "N" {
      }
      frame "S" {
      }
    }
    n441 = case shown="\"O\", Default" w521 {
      tunnel: [0 1 2] -> w520
      frame "O", Default {
      }
      frame "R" {
      }
      frame "L" {
      }
    }
    n442 = To Long Integer(number=w554) -> (32bit integer=w600:i32)
    n443 = case shown="\"O\", Default" w483 {
      tunnel: [0 1 2] -> w518
      frame "O", Default {
      }
      frame "I" {
      }
      frame "M" {
      }
    }
    n444 = Format Into String(format string="%d", w502) -> (resulting string=w532:string)  [unwired: 2 in, 1 out]
    n445 = Format Into String(format string="%03d", w600) -> (resulting string=w488:string)  [unwired: 2 in, 1 out]
    n446 = Format Into String(format string="%d", w494) -> (resulting string=w561:string)  [unwired: 2 in, 1 out]
    n447 = Not Equal To 0?(x=w511) -> (x != 0?=w510:bool)
    n448 = local read "False Alarm"() -> (w493:bool)
    n449 = Build Array(w511, w520, w519, w518) -> (w509:i32[])
    n450 = case shown="True" w510 {
      tunnel: w509 -> [_ w633]
      tunnel: w482 -> [_ _]
      frame False {
      }
      frame True {
        "StimInfo" <- w633
      }
    }
    n451 = Boolean To (0,1)(Boolean=w493) -> (0, 1=w492:i16)
    n452 = Tick Count (ms)() -> (millisecond timer value=w586:u32)
    n453 = call "Elapsed Time"("Time Target (s)"=w586) -> ("Elapsed Time (s)"=w541:dbl)  [unwired: 11 in, 7 out]
    "Elapsed Time" <- w541
    n454 = Format Into String(format string="%d", w492) -> (resulting string=w489:string)  [unwired: 2 in, 1 out]
    n455 = local read "StimInfo"() -> (w480:i32[])
    n456 = Concatenate Strings(w561, w563, w501, w532, w489, w488, w490) -> (w575:string)
    n457 = Or(x=w607, y=w536) -> (x .or. y?=w590:bool)
    "Correct" <- w590
    n458 = Build Array (concatenate)(w480, w479) -> (w478:i32[])
    n459 = To Single Precision Float(number=w478) -> (single precision float=w517:sgl[])
    n460 = To Single Precision Float(number=w494) -> (single precision float=w610:sgl)
    n461 = Boolean To (0,1)(Boolean=w614) -> (0, 1=w613:i16)
    n462 = Boolean To (0,1)(Boolean=w536) -> (0, 1=w612:i16)
    n463 = To Single Precision Float(number=w613) -> (single precision float=w609:sgl)
    n464 = call-poly <vilib>:"DAQmx Write.vi"("task/channels in"=w595, "data"=w590, "timeout"=1.0) -> ("task out"=w597:refnum<k21>, "error out"=w596:errorcluster)  [unwired: 10 in, 1 out]
    n465 = To Single Precision Float(number=w612) -> (single precision float=w608:sgl)
    n466 = Lossy Enqueue Element(queue=w585, element=w541, error in (no error)=w584) -> ()  [unwired: 4 out]
    n467 = Build Array (concatenate)(w551, w610, w609, w608, w611, w517) -> (w587:sgl[])
    n468 = local read "File Open"() -> (w583:bool)
    n469 = local read "Encoder Ref Out"() -> (w582:refnum<file>)
    n470 = call <vilib>:"DAQmx Start Task.vi"("task/channels in"=w597, "error in"=w596) -> ("task out"=w594:refnum<k21>, "error out"=w593:errorcluster)  [unwired: 12 in]
    n471 = case shown="True" w583 {
      tunnel: [w728 w734] -> _
      tunnel: [w727 w733] -> _
      tunnel: w582 -> [w719 w731]
      tunnel: w587 -> [w720 w730]
      tunnel: w541 -> [w721 w729]
      frame False {
        w722 = FALSE ("prepend array or string size? (T)")
        n472 = Write to Binary File(file (use dialog)=w719, data=w720, 5:w722) -> (refnum out=w726:refnum<file>, error out=w725:errorcluster)  [unwired: 3 in, 1 out]
        n473 = Write to Binary File(file (use dialog)=w726, data=w721, error in=w725, 5:w722) -> (refnum out=w723:refnum<file>, error out=w724:errorcluster)  [unwired: 2 in, 1 out]
        n474 = Flush File(refnum=w723, error in=w724) -> (refnum out=w728:refnum<file>, error out=w727:errorcluster)
      }
      frame True {
        w732 = FALSE ("prepend array or string size? (T)")
        n475 = Write to Binary File(file (use dialog)=w731, data=w730, 5:w732) -> (refnum out=w736:refnum<file>, error out=w735:errorcluster)  [unwired: 3 in, 1 out]
        n476 = Write to Binary File(file (use dialog)=w736, data=w729, error in=w735, 5:w732) -> (refnum out=w734:refnum<file>, error out=w733:errorcluster)  [unwired: 2 in, 1 out]
        "Encoder\n Ref Out 2" <- w734
      }
    }
    n477 = String To IP(1:"169.230.68.195" ("name")) -> (0:w576:u32)
    n478 = property on="SAVE" class="Bool (strict)"() -> ("Value"=w542:bool)  [unwired: 2 in, 2 out]
    n479 = UDP Write(address=w576, port or service name=u16 8888 ("Remote Port"), connection ID=w574, data in=w575, 8:w573, 9:1000 ("timeout ms (25000)")) -> (error out=w571:errorcluster, 3:w572:refnum<k16>)
    n480 = case shown="True" w542 {
      tunnel: w541 -> [_ w652]
      frame False {
        (unwired) FALSE
        n481 = local read "Save Time Start"() -> (w650:bool)
        n482 = case shown="True" w650 {
          frame False {
          }
          frame True {
            w651 = TRUE
            n483 = property on="SAVE" class="Bool (strict)"("Val(Sgnl)"=w651) -> ()  [unwired: 2 in, 2 out]
            n484 = property on="SAVE" class="Bool (strict)"("Value"=w651) -> ()  [unwired: 2 in, 2 out]
          }
        }
      }
      frame True {
        n485 = local read "Save Time Start"() -> (w653:bool)
        n486 = case shown="True" w653 {
          tunnel: w652 -> [w654 w657]
          frame False {
            (unwired) FALSE
            "Save Time Start" <- TRUE ("Close All")
            "Save Start Time" <- w654
          }
          frame True {
            w661 = 600.0 ("y")
            n487 = local read "Save Start Time"() -> (w658:dbl)
            n488 = Subtract(x=w657, y=w658) -> (x-y=w659:dbl)
            n489 = Quotient & Remainder(x=w659, y=w661) -> (x-y*floor(x/y)=w660:dbl)  [unwired: 1 out]
            n490 = Subtract(x=w661, y=0.1) -> (x-y=w663:dbl)
            n491 = Greater?(x=w660, y=w663) -> (0:w656:bool)
            n492 = case shown="True" w656 {
              frame False {
              }
              frame True {
                w664 = FALSE ("SAVE ALL")
                n493 = property on="SAVE" class="Bool (strict)"("Val(Sgnl)"=w664) -> ()  [unwired: 2 in, 2 out]
                n494 = property on="SAVE" class="Bool (strict)"("Value"=w664) -> ()  [unwired: 2 in, 2 out]
              }
            }
          }
        }
      }
    }
    n495 = node-c288() -> ()  [unwired: 1 in, 1 out]
    "Timer Q Out" <- w585
    "Numeric" <- w516
  }
  n496 = call-poly <vilib>:"DAQmx Write.vi"("task/channels in"=w40, "data"=FALSE, "error in"=w39) -> ("task out"=w50:refnum<k21>, "error out"=w49:errorcluster)  [unwired: 10 in, 1 out]
  n497 = call <vilib>:"DAQmx Clear Task.vi"("task in"=w50, "error in"=w49) -> ()  [unwired: 13 in, 1 out]
  n498 = Get Date/Time String(date format (0)=enum16{"short", "long", "abbreviated"}."long", want seconds? (F)=TRUE) -> (date string=w64:string, time string=w66:string)  [unwired: 1 in]
  n499 = Search and Replace String(input string=w66, search string=":") -> (result string=w71:string, error out=w62:errorcluster)  [unwired: 6 in, 2 out]
  n500 = Search and Replace String(input string=w71, search string=":", replace string=" " ("replace string (\"\")"), error in=w62) -> (result string=w72:string)  [unwired: 4 in, 3 out]
  n501 = call <vilib>:"Space Constant.vi"() -> ("String"=w65:string)
  n502 = Concatenate Strings("E:\\Data\\BH\\" ("Image Name"), "Mouse Name", "\\" ("replace string (\"\")"), w64, w65, w72) -> (w58:string)
  n503 = String To Path(string=w58) -> (path=w55:path)
  n504 = call <vilib>:"Check if File or Folder Exists.vi"("path"=w55) -> ("file or folder exists?"=w57:bool, "dup path"=w56:path)  [unwired: 8 in, 1 out]
  n505 = call <vilib>:"TCP Listen.vi"("timeout ms (wait forever: -1)"=-1, "port"="Port") -> ("error out"=w101:errorcluster, "connection ID"=w102:refnum<k5>)  [unwired: 5 in, 3 out]
  n506 = case shown="True" w57 {
    tunnel: [w1160 w1161] -> w54
    tunnel: w56 -> [w1159 w1161]
    frame False {
      n507 = Create Folder(path (use dialog)=w1159) -> (created path=w1160:path)  [unwired: 2 in, 2 out]
    }
    frame True {
    }
  }
  "File Save Path" <- w54
  n508 = case shown="No Error" w101 {
    selector: w101 -> [_ w1856]
    tunnel: [w1167 w1856] -> w106
    tunnel: w102 -> [w1172 w1857]
    tunnel: [w1172 w1857] -> w107
    tunnel: [FALSE FALSE] -> w105
    frame No Error {
      w1166 = 56 items=["No Error", "Argument Error", "Memory Full", "Out of Zone", "End of File", "File Already Open", "Generic File IO Error", "File Not Found", "File Permission Error", "Disk Full", "Duplicate Path", "Too Many Files Open", "Not Enabled", "Resource File Not Found", "Cannot Add Resource", "Resource Not Found", "Image Not Found", "Image Memory Error", "Pen Does Not Exist", "Config Bad Type", "Config Token Not Found", "Config Parse Error", "Config Memory Error", "Bad External Code Format", "Bad External Code Offset", "External Code Not Present", "Null Window", "Destroy Window Mixup", "Null Menu", "Print Aborted", "Bad Print Record", "Print Driver Error", "Windows Error During Print", "Memory Error During Print", "Print Dialog Error", "Generic Print Error", "Invalid Device Refnum", "Device Not Found", "Device Parameter Error", "Device Unit Error", "Can't Open Device", "Device Call Aborted", "Generic Error", "Cancelled By User", "Object ID Too Low", "Object ID Too High", "Object Not In Heap", "Unknown Heap", "Bad DefProc ID", "DefProc Not In Table", "Message Out Of Range", "Null Method", "Unknown Message", "Manager Call Not Supported", "Bad address", "Connection In progress", "Connection timed out", "Connection is already in progress", "Network attribute not supported", "Network error", "Address in use", "System out of memory", "Connection aborted", "Connection refused", "Connection is not connected", "Connection is already connected", "Connection closed", "Initialize error (interapplication manager)", "Bad occurrence", "Wait on unbound occurrence handler", "Occurrence queue overflow", "Bad path", "Semaphore not signaled", "Unrecognized type (interapplication manager)"] ("2nd Error to Convert")
      w1168 = 66 items=["No Error", "Argument Error", "Memory Full", "Out of Zone", "End of File", "File Already Open", "Generic File IO Error", "File Not Found", "File Permission Error", "Disk Full", "Duplicate Path", "Too Many Files Open", "Not Enabled", "Resource File Not Found", "Cannot Add Resource", "Resource Not Found", "Image Not Found", "Image Memory Error", "Pen Does Not Exist", "Config Bad Type", "Config Token Not Found", "Config Parse Error", "Config Memory Error", "Bad External Code Format", "Bad External Code Offset", "External Code Not Present", "Null Window", "Destroy Window Mixup", "Null Menu", "Print Aborted", "Bad Print Record", "Print Driver Error", "Windows Error During Print", "Memory Error During Print", "Print Dialog Error", "Generic Print Error", "Invalid Device Refnum", "Device Not Found", "Device Parameter Error", "Device Unit Error", "Can't Open Device", "Device Call Aborted", "Generic Error", "Cancelled By User", "Object ID Too Low", "Object ID Too High", "Object Not In Heap", "Unknown Heap", "Bad DefProc ID", "DefProc Not In Table", "Message Out Of Range", "Null Method", "Unknown Message", "Manager Call Not Supported", "Bad address", "Connection In progress", "Connection timed out", "Connection is already in progress", "Network attribute not supported", "Network error", "Address in use", "System out of memory", "Connection aborted", "Connection refused", "Connection is not connected", "Connection is already connected", "Connection closed", "Initialize error (interapplication manager)", "Bad occurrence", "Wait on unbound occurrence handler", "Occurrence queue overflow", "Bad path", "Semaphore not signaled", "Unrecognized type (interapplication manager)"] ("3rd Error to Convert")
      w1169 = 64 items=["No Error", "Argument Error", "Memory Full", "Out of Zone", "End of File", "File Already Open", "Generic File IO Error", "File Not Found", "File Permission Error", "Disk Full", "Duplicate Path", "Too Many Files Open", "Not Enabled", "Resource File Not Found", "Cannot Add Resource", "Resource Not Found", "Image Not Found", "Image Memory Error", "Pen Does Not Exist", "Config Bad Type", "Config Token Not Found", "Config Parse Error", "Config Memory Error", "Bad External Code Format", "Bad External Code Offset", "External Code Not Present", "Null Window", "Destroy Window Mixup", "Null Menu", "Print Aborted", "Bad Print Record", "Print Driver Error", "Windows Error During Print", "Memory Error During Print", "Print Dialog Error", "Generic Print Error", "Invalid Device Refnum", "Device Not Found", "Device Parameter Error", "Device Unit Error", "Can't Open Device", "Device Call Aborted", "Generic Error", "Cancelled By User", "Object ID Too Low", "Object ID Too High", "Object Not In Heap", "Unknown Heap", "Bad DefProc ID", "DefProc Not In Table", "Message Out Of Range", "Null Method", "Unknown Message", "Manager Call Not Supported", "Bad address", "Connection In progress", "Connection timed out", "Connection is already in progress", "Network attribute not supported", "Network error", "Address in use", "System out of memory", "Connection aborted", "Connection refused", "Connection is not connected", "Connection is already connected", "Connection closed", "Initialize error (interapplication manager)", "Bad occurrence", "Wait on unbound occurrence handler", "Occurrence queue overflow", "Bad path", "Semaphore not signaled", "Unrecognized type (interapplication manager)"] ("1st Error to Convert")
      n509 = while "Send loop" {
        tunnel: w1172 -> [w1193]
        tunnel: [w1195] -> w1163
        tunnel: [w1192] -> w1171
        shift-left: "" -> [w1196]
        shift-right: [w1194] -> _
        tunnel: [w1174] -> w1162
        stop <- w1195 stop-if-true
        w1185 = 10000 ("y")
        n510 = local read "Input Line"() -> (w1175:string)
        n511 = case shown="\"SqrGrtPtch 2\"" "Tab Control" {
          tunnel: [w1198 w1216 w1232 w1248 w1251 w1267 w1288 w1297 w1330 w1346 w1375 w1378 w1387 w1406 w1422 w1454 w1481 w1510 w1523 w1573 w1585 w1618 w1636 w1647 w1664 w1697 w1710 w1729 w1747 w1772 w1790 w1823] -> w1182
          frame "Barnoise", Default {
            # "don't clear"
            # "synctoVBL"
            n512 = Number To Decimal String(number="Rects per height") -> (decimal integer string=w1204:string)  [unwired: 1 in]
            n513 = Number To Decimal String(number="Rects per width") -> (decimal integer string=w1203:string)  [unwired: 1 in]
            n514 = Number To Decimal String(number="Scaling factor") -> (decimal integer string=w1202:string)  [unwired: 1 in]
            n515 = Number To Decimal String(number=1) -> (decimal integer string=w1201:string)  [unwired: 1 in]
            n516 = Number To Decimal String(number=0) -> (decimal integer string=w1200:string)  [unwired: 1 in]
            n517 = Number To Decimal String(number="Stimlength (s)") -> (decimal integer string=w1199:string)  [unwired: 1 in]
            n518 = Number To Decimal String(number=1) -> (decimal integer string=w1205:string)  [unwired: 1 in]
            n519 = call <vilib>:"Space Constant.vi"() -> ("String"=w1206:string)
            n520 = Concatenate Strings(w1205, w1206, w1204, w1206, w1203, w1206, w1202, w1206, w1201, w1206, w1200, w1206, w1199) -> (w1198:string)
          }
          frame "Circle" {
            n521 = Number To Decimal String(number="radius") -> (decimal integer string=w1219:string)  [unwired: 1 in]
            n522 = Number To Decimal String(number="interval (s)") -> (decimal integer string=w1218:string)  [unwired: 1 in]
            n523 = Number To Decimal String(number="# of circles") -> (decimal integer string=w1217:string)  [unwired: 1 in]
            n524 = Number To Decimal String(number="# of flashes/circles") -> (decimal integer string=w1213:string)  [unwired: 1 in]
            n525 = Number To Decimal String(number=3) -> (decimal integer string=w1220:string)  [unwired: 1 in]
            n526 = call <vilib>:"Space Constant.vi"() -> ("String"=w1214:string)
            n527 = Concatenate Strings(w1220, w1214, w1219, w1214, w1218, w1214, w1217, w1214, w1213) -> (w1216:string)
          }
          frame "driftgrat" {
            n528 = Number To Decimal String(number="cycles per second") -> (decimal integer string=w1234:string)  [unwired: 1 in]
            n529 = Number To Decimal String(number=11) -> (decimal integer string=w1237:string)  [unwired: 1 in]
            n530 = Number To Decimal String(number="period") -> (decimal integer string=w1233:string)  [unwired: 1 in]
            n531 = Number To Decimal String(number="duration") -> (decimal integer string=w1231:string)  [unwired: 1 in]
            n532 = Number To Decimal String(number="repeats") -> (decimal integer string=w1230:string)  [unwired: 1 in]
            n533 = Number To Decimal String(number="amplitude") -> (decimal integer string=w1228:string)  [unwired: 1 in]
            n534 = call <vilib>:"Space Constant.vi"() -> ("String"=w1229:string)
            n535 = Concatenate Strings(w1237, w1229, w1234, w1229, w1233, w1229, w1231, w1229, w1230, w1229, w1228) -> (w1232:string)
          }
          frame "whitebar" {
            n536 = Number To Decimal String(number="line width") -> (decimal integer string=w1246:string)  [unwired: 1 in]
            n537 = Number To Decimal String(number="x velocity") -> (decimal integer string=w1244:string)  [unwired: 1 in]
            n538 = Number To Decimal String(number="y velocity") -> (decimal integer string=w1243:string)  [unwired: 1 in]
            n539 = Number To Decimal String(number="repeats 2") -> (decimal integer string=w1239:string)  [unwired: 1 in]
            n540 = Number To Decimal String(number=10) -> (decimal integer string=w1249:string)  [unwired: 1 in]
            n541 = call <vilib>:"Space Constant.vi"() -> ("String"=w1240:string)
            n542 = Concatenate Strings(w1249, w1240, w1246, w1240, w1244, w1240, w1243, w1240, w1239) -> (w1248:string)
          }
          frame "spotramp" {
            n543 = Number To Decimal String(number="Xcenter") -> (decimal integer string=w1259:string)  [unwired: 1 in]
            n544 = Number To Decimal String(number="repeats 7") -> (decimal integer string=w1257:string)  [unwired: 1 in]
            n545 = Number To Decimal String(number="radius 4") -> (decimal integer string=w1256:string)  [unwired: 1 in]
            n546 = Number To Decimal String(number="duration 2") -> (decimal integer string=w1255:string)  [unwired: 1 in]
            n547 = Number To Decimal String(number="increment") -> (decimal integer string=w1252:string)  [unwired: 1 in]
            n548 = Number To Decimal String(number="Ycenter") -> (decimal integer string=w1258:string)  [unwired: 1 in]
            n549 = Number To Decimal String(number=20) -> (decimal integer string=w1260:string)  [unwired: 1 in]
            n550 = call <vilib>:"Space Constant.vi"() -> ("String"=w1254:string)
            n551 = Concatenate Strings(w1260, w1254, w1259, w1254, w1258, w1254, w1257, w1254, w1256, w1254, w1255, w1254, w1252, w1254) -> (w1251:string)
          }
          frame "flickerspots" {
            n552 = local read "number (0 to 1) 2"() -> (w1274:dbl)
            n553 = Number To Decimal String(number="1on 2off 3 onoff") -> (decimal integer string=w1279:string)  [unwired: 1 in]
            n554 = Number To Decimal String(number="duration 4") -> (decimal integer string=w1277:string)  [unwired: 1 in]
            n555 = Number To Decimal String(number="gridsize") -> (decimal integer string=w1276:string)  [unwired: 1 in]
            n556 = Number To Decimal String(number="repeats 8") -> (decimal integer string=w1278:string)  [unwired: 1 in]
            n557 = Multiply(x=w1274, y=100000.0) -> (x*y=w1272:dbl)
            n558 = Number To Decimal String(number="spotsperflash") -> (decimal integer string=w1268:string)  [unwired: 1 in]
            n559 = Number To Decimal String(number=21) -> (decimal integer string=w1280:string)  [unwired: 1 in]
            n560 = call <vilib>:"Space Constant.vi"() -> ("String"=w1270:string)
            n561 = To Long Integer(number=w1272) -> (32bit integer=w1275:i32)
            "randinput 3" <- w1275
            n562 = Number To Decimal String(number=w1275) -> (decimal integer string=w1271:string)  [unwired: 1 in]
            n563 = Concatenate Strings(w1280, w1270, w1279, w1270, w1278, w1270, w1277, w1270, w1276, w1270, w1271, w1270, w1268, w1270) -> (w1267:string)
          }
          frame "Ring" {
            n564 = Number To Decimal String(number="ring width") -> (decimal integer string=w1292:string)  [unwired: 1 in]
            n565 = Number To Decimal String(number="# of flashes/ring") -> (decimal integer string=w1290:string)  [unwired: 1 in]
            n566 = Number To Decimal String(number="interval 2 (ms)", width (-)=i16 3) -> (decimal integer string=w1291:string)
            n567 = Number To Decimal String(number=2) -> (decimal integer string=w1293:string)  [unwired: 1 in]
            n568 = call <vilib>:"Space Constant.vi"() -> ("String"=w1289:string)
            n569 = Concatenate Strings(w1293, w1289, w1292, w1289, w1291, w1289, w1290) -> (w1288:string)
          }
          frame "switchgrate" {
            n570 = Number To Decimal String(number="period 2") -> (decimal integer string=w1309:string)  [unwired: 1 in]
            n571 = Number To Decimal String(number="repeats 5") -> (decimal integer string=w1308:string)  [unwired: 1 in]
            n572 = Number To Decimal String(number="rotation") -> (decimal integer string=w1306:string)  [unwired: 1 in]
            n573 = Number To Decimal String(number="radius 3") -> (decimal integer string=w1305:string)  [unwired: 1 in]
            n574 = Number To Decimal String(number="xcenter") -> (decimal integer string=w1304:string)  [unwired: 1 in]
            n575 = Number To Decimal String(number="ycenter") -> (decimal integer string=w1299:string)  [unwired: 1 in]
            n576 = Number To Decimal String(number="background 2") -> (decimal integer string=w1301:string)  [unwired: 1 in]
            n577 = Number To Decimal String(number="period in pixels", width (-)=i16 3) -> (decimal integer string=w1307:string)
            n578 = Number To Decimal String(number=18) -> (decimal integer string=w1310:string)  [unwired: 1 in]
            n579 = call <vilib>:"Space Constant.vi"() -> ("String"=w1300:string)
            n580 = Concatenate Strings(w1310, w1300, w1309, w1300, w1308, w1300, w1307, w1300, w1306, w1300, w1305, w1300, w1304, w1300, w1299, w1300, w1301) -> (w1297:string)
          }
          frame "loom" {
            n581 = Number To Decimal String(number="ringR") -> (decimal integer string=w1342:string)  [unwired: 1 in]
            n582 = Number To Decimal String(number="speed") -> (decimal integer string=w1341:string)  [unwired: 1 in]
            n583 = Number To Decimal String(number="msinterval") -> (decimal integer string=w1340:string)  [unwired: 1 in]
            n584 = Number To Decimal String(number="repeats 3") -> (decimal integer string=w1339:string)  [unwired: 1 in]
            n585 = Number To Decimal String(number="centerx") -> (decimal integer string=w1334:string)  [unwired: 1 in]
            n586 = Number To Decimal String(number="bool") -> (decimal integer string=w1326:string)  [unwired: 1 in]
            n587 = Number To Decimal String(number="backg") -> (decimal integer string=w1331:string)  [unwired: 1 in]
            n588 = Number To Decimal String(number="blanktime") -> (decimal integer string=w1324:string)  [unwired: 1 in]
            n589 = Number To Decimal String(number="centery") -> (decimal integer string=w1332:string)  [unwired: 1 in]
            n590 = call <vilib>:"Space Constant.vi"() -> ("String"=w1323:string)
            n591 = local read "number (0 to 1) 2"() -> (w1321:dbl)
            n592 = Number To Decimal String(number=17) -> (decimal integer string=w1328:string)  [unwired: 1 in]
            n593 = Multiply(x=w1321, y=100000.0) -> (x*y=w1319:dbl)
            n594 = To Long Integer(number=w1319) -> (32bit integer=w1322:i32)
            "randinput" <- w1322
            n595 = Number To Decimal String(number=w1322) -> (decimal integer string=w1318:string)  [unwired: 1 in]
            n596 = Concatenate Strings(w1328, w1323, w1342, w1323, w1341, w1323, w1340, w1323, w1339, w1323, w1334, w1323, w1332, w1323, w1331, w1323, w1326, w1323, w1324, w1323, w1318, w1323) -> (w1330:string)
          }
          frame "pinwheel" {
            n597 = Number To Decimal String(number="bar radius") -> (decimal integer string=w1369:string)  [unwired: 1 in]
            n598 = Number To Decimal String(number="speed 2") -> (decimal integer string=w1368:string)  [unwired: 1 in]
            n599 = Number To Decimal String(number="msinterval 6") -> (decimal integer string=w1367:string)  [unwired: 1 in]
            n600 = Number To Decimal String(number="repeats 18") -> (decimal integer string=w1366:string)  [unwired: 1 in]
            n601 = Number To Decimal String(number="centerx 2") -> (decimal integer string=w1361:string)  [unwired: 1 in]
            n602 = Number To Decimal String(number="0 for bar \n1 for cross") -> (decimal integer string=w1354:string)  [unwired: 1 in]
            n603 = Number To Decimal String(number="backg 5") -> (decimal integer string=w1358:string)  [unwired: 1 in]
            n604 = Number To Decimal String(number="blanktime 2") -> (decimal integer string=w1352:string)  [unwired: 1 in]
            n605 = Number To Decimal String(number="centery 2") -> (decimal integer string=w1359:string)  [unwired: 1 in]
            n606 = call <vilib>:"Space Constant.vi"() -> ("String"=w1351:string)
            n607 = local read "number (0 to 1) 2"() -> (w1349:dbl)
            n608 = Number To Decimal String(number=30) -> (decimal integer string=w1356:string)  [unwired: 1 in]
            n609 = Multiply(x=w1349, y=100000.0) -> (x*y=w1347:dbl)
            n610 = To Long Integer(number=w1347) -> (32bit integer=w1350:i32)
            "randinput 5" <- w1350
            n611 = Number To Decimal String(number=w1350) -> (decimal integer string=w1345:string)  [unwired: 1 in]
            n612 = Concatenate Strings(w1356, w1351, w1369, w1351, w1368, w1351, w1367, w1351, w1366, w1351, w1361, w1351, w1359, w1351, w1358, w1351, w1354, w1351, w1352, w1351, w1345, w1351) -> (w1346:string)
          }
          frame "Probe" {
            n613 = Number To Decimal String(number="spot intensity") -> (decimal integer string=w1373:string)  [unwired: 1 in]
            n614 = Number To Decimal String(number=4) -> (decimal integer string=w1376:string)  [unwired: 1 in]
            n615 = call <vilib>:"Space Constant.vi"() -> ("String"=w1372:string)
            n616 = Concatenate Strings(w1376, w1372, w1373) -> (w1375:string)
          }
          frame "fullfieldonoff" {
            n617 = Number To Decimal String(number="# of flashes") -> (decimal integer string=w1381:string)  [unwired: 1 in]
            n618 = Number To Decimal String(number=14) -> (decimal integer string=w1384:string)  [unwired: 1 in]
            n619 = Number To Decimal String(number="flash frame length") -> (decimal integer string=w1380:string)  [unwired: 1 in]
            n620 = call <vilib>:"Space Constant.vi"() -> ("String"=w1379:string)
            n621 = Concatenate Strings(w1384, w1379, w1381, w1379, w1380) -> (w1378:string)
          }
          frame "Moving bar" {
            n622 = Number To Decimal String(number="Velocity (pix/s)") -> (decimal integer string=w1391:string)  [unwired: 1 in]
            n623 = Number To Decimal String(number="Length (pixels)") -> (decimal integer string=w1390:string)  [unwired: 1 in]
            n624 = Number To Decimal String(number="Width (pixels)") -> (decimal integer string=w1389:string)  [unwired: 1 in]
            n625 = Number To Decimal String(number="repeats 4") -> (decimal integer string=w1388:string)  [unwired: 1 in]
            n626 = Number To Decimal String(number=5) -> (decimal integer string=w1392:string)  [unwired: 1 in]
            n627 = call <vilib>:"Space Constant.vi"() -> ("String"=w1386:string)
            n628 = Concatenate Strings(w1392, w1386, w1391, w1386, w1390, w1386, w1389, w1386, w1388, w1386) -> (w1387:string)
          }
          frame "OMS" {
            n629 = Number To Decimal String(number="Background\nangle") -> (decimal integer string=w1412:string)  [unwired: 1 in]
            n630 = Number To Decimal String(number="Background\ncycles/s") -> (decimal integer string=w1411:string)  [unwired: 1 in]
            n631 = Number To Decimal String(number="Object angle") -> (decimal integer string=w1409:string)  [unwired: 1 in]
            n632 = Number To Decimal String(number="Object size") -> (decimal integer string=w1408:string)  [unwired: 1 in]
            n633 = Number To Decimal String(number="Object phase") -> (decimal integer string=w1407:string)  [unwired: 1 in]
            n634 = Number To Decimal String(number="Global time") -> (decimal integer string=w1399:string)  [unwired: 1 in]
            n635 = Number To Decimal String(number="Differential time") -> (decimal integer string=w1401:string)  [unwired: 1 in]
            n636 = Number To Decimal String(number="Local time") -> (decimal integer string=w1402:string)  [unwired: 1 in]
            n637 = Number To Decimal String(number="Background\nspatial frequency", width (-)=i16 3) -> (decimal integer string=w1410:string)
            n638 = Number To Decimal String(number=6) -> (decimal integer string=w1413:string)  [unwired: 1 in]
            n639 = call <vilib>:"Space Constant.vi"() -> ("String"=w1400:string)
            n640 = Concatenate Strings(w1413, w1400, w1412, w1400, w1411, w1400, w1410, w1400, w1409, w1400, w1408, w1400, w1407, w1400, w1399, w1400, w1401, w1400, w1402) -> (w1406:string)
          }
          frame "newloom" {
            n641 = Number To Decimal String(number="xcenter 2") -> (decimal integer string=w1443:string)  [unwired: 1 in]
            n642 = Number To Decimal String(number="ycenter 2") -> (decimal integer string=w1442:string)  [unwired: 1 in]
            n643 = Number To Decimal String(number="repeats 6") -> (decimal integer string=w1441:string)  [unwired: 1 in]
            n644 = Number To Decimal String(number="rate") -> (decimal integer string=w1440:string)  [unwired: 1 in]
            n645 = Number To Decimal String(number="initRadius") -> (decimal integer string=w1435:string)  [unwired: 1 in]
            n646 = Number To Decimal String(number="msinterval 2") -> (decimal integer string=w1432:string)  [unwired: 1 in]
            n647 = Number To Decimal String(number="grayDelay") -> (decimal integer string=w1428:string)  [unwired: 1 in]
            n648 = Number To Decimal String(number="msDelay") -> (decimal integer string=w1433:string)  [unwired: 1 in]
            n649 = call <vilib>:"Space Constant.vi"() -> ("String"=w1427:string)
            n650 = local read "number (0 to 1) 2"() -> (w1425:dbl)
            n651 = Number To Decimal String(number=19) -> (decimal integer string=w1430:string)  [unwired: 1 in]
            n652 = Multiply(x=w1425, y=100000.0) -> (x*y=w1423:dbl)
            n653 = To Long Integer(number=w1423) -> (32bit integer=w1426:i32)
            "randinput 2" <- w1426
            n654 = Number To Decimal String(number=w1426) -> (decimal integer string=w1421:string)  [unwired: 1 in]
            n655 = Concatenate Strings(w1430, w1427, w1443, w1427, w1442, w1427, w1441, w1427, w1440, w1427, w1435, w1427, w1433, w1427, w1432, w1427, w1421, w1427, w1428, w1427) -> (w1422:string)
          }
          frame "distractor" {
            n656 = Number To Decimal String(number="xcenter 3") -> (decimal integer string=w1474:string)  [unwired: 1 in]
            n657 = Number To Decimal String(number="ycenter 3") -> (decimal integer string=w1473:string)  [unwired: 1 in]
            n658 = Number To Decimal String(number="repeats 10") -> (decimal integer string=w1472:string)  [unwired: 1 in]
            n659 = Number To Decimal String(number="rate 2") -> (decimal integer string=w1471:string)  [unwired: 1 in]
            n660 = Number To Decimal String(number="initRadius 2") -> (decimal integer string=w1466:string)  [unwired: 1 in]
            n661 = Number To Decimal String(number="msinterval 3") -> (decimal integer string=w1463:string)  [unwired: 1 in]
            n662 = Number To Decimal String(number="grayDelay 2") -> (decimal integer string=w1460:string)  [unwired: 1 in]
            n663 = Number To Decimal String(number="msDelay 2") -> (decimal integer string=w1464:string)  [unwired: 1 in]
            n664 = call <vilib>:"Space Constant.vi"() -> ("String"=w1448:string)
            n665 = local read "number (0 to 1) 2"() -> (w1458:dbl)
            n666 = Number To Decimal String(number=23) -> (decimal integer string=w1462:string)  [unwired: 1 in]
            n667 = Multiply(x=w1458, y=100000.0) -> (x*y=w1456:dbl)
            n668 = To Long Integer(number=w1456) -> (32bit integer=w1459:i32)
            "randinput 4" <- w1459
            n669 = Number To Decimal String(number="dxcenter") -> (decimal integer string=w1450:string)  [unwired: 1 in]
            n670 = Number To Decimal String(number="dycenter") -> (decimal integer string=w1449:string)  [unwired: 1 in]
            n671 = Number To Decimal String(number="offsetms") -> (decimal integer string=w1446:string)  [unwired: 1 in]
            n672 = Number To Decimal String(number=w1459) -> (decimal integer string=w1455:string)  [unwired: 1 in]
            n673 = Concatenate Strings(w1462, w1448, w1474, w1448, w1473, w1448, w1472, w1448, w1471, w1448, w1466, w1448, w1464, w1448, w1463, w1448, w1455, w1448, w1460, w1448, w1450, w1448, w1449, w1448, w1446, w1448) -> (w1454:string)
          }
          frame "Rasterspot" {
            n674 = Number To Decimal String(number="radius 2") -> (decimal integer string=w1486:string)  [unwired: 1 in]
            n675 = Number To Decimal String(number="# of x spots") -> (decimal integer string=w1484:string)  [unwired: 1 in]
            n676 = Number To Decimal String(number="# of y spots") -> (decimal integer string=w1483:string)  [unwired: 1 in]
            n677 = Number To Decimal String(number="# of flashes/spot") -> (decimal integer string=w1482:string)  [unwired: 1 in]
            n678 = Number To Decimal String(number="repeats 9") -> (decimal integer string=w1477:string)  [unwired: 1 in]
            n679 = Number To Decimal String(number="time interval (ms)", width (-)=i16 3) -> (decimal integer string=w1485:string)
            n680 = Number To Decimal String(number=7) -> (decimal integer string=w1487:string)  [unwired: 1 in]
            n681 = call <vilib>:"Space Constant.vi"() -> ("String"=w1479:string)
            n682 = Concatenate Strings(w1487, w1479, w1486, w1479, w1485, w1479, w1484, w1479, w1483, w1479, w1482, w1479, w1477, w1479) -> (w1481:string)
          }
          frame "Screenchop" {
            n683 = local read "number (0 to 1) 2"() -> (w1508:dbl)
            n684 = Number To Decimal String(number="chopx") -> (decimal integer string=w1518:string)  [unwired: 1 in]
            n685 = Number To Decimal String(number=15) -> (decimal integer string=w1521:string)  [unwired: 1 in]
            n686 = Number To Decimal String(number="chopy") -> (decimal integer string=w1517:string)  [unwired: 1 in]
            n687 = Number To Decimal String(number="msinterval 4") -> (decimal integer string=w1516:string)  [unwired: 1 in]
            n688 = Number To Decimal String(number="flashnum") -> (decimal integer string=w1515:string)  [unwired: 1 in]
            n689 = Number To Decimal String(number="repeats  11") -> (decimal integer string=w1514:string)  [unwired: 1 in]
            n690 = Number To Decimal String(number="grayframes") -> (decimal integer string=w1503:string)  [unwired: 1 in]
            n691 = Number To Decimal String(number="flashbrightness") -> (decimal integer string=w1501:string)  [unwired: 1 in]
            n692 = call <vilib>:"Space Constant.vi"() -> ("String"=w1498:string)
            n693 = Multiply(x=w1508, y=100000.0) -> (x*y=w1506:dbl)
            n694 = To Long Integer(number=w1506) -> (32bit integer=w1509:i32)
            "seed  1" <- w1509
            n695 = Number To Decimal String(number="boxsize") -> (decimal integer string=w1500:string)  [unwired: 1 in]
            n696 = Number To Decimal String(number=w1509) -> (decimal integer string=w1505:string)  [unwired: 1 in]
            n697 = Number To Decimal String(number="xcenter 4") -> (decimal integer string=w1497:string)  [unwired: 1 in]
            n698 = Number To Decimal String(number="ycenter 4") -> (decimal integer string=w1494:string)  [unwired: 1 in]
            n699 = Concatenate Strings(w1521, w1498, w1518, w1498, w1517, w1498, w1516, w1498, w1515, w1498, w1514, w1498, w1505, w1498, w1503, w1498, w1501, w1498, w1500, w1498, w1497, w1498, w1494, w1498) -> (w1510:string)
          }
          frame "Screenchopbars" {
            n700 = local read "number (0 to 1) 2"() -> (w1538:dbl)
            n701 = Number To Decimal String(number="chopx 2") -> (decimal integer string=w1547:string)  [unwired: 1 in]
            n702 = Number To Decimal String(number=25) -> (decimal integer string=w1550:string)  [unwired: 1 in]
            n703 = Number To Decimal String(number="chopy 2") -> (decimal integer string=w1546:string)  [unwired: 1 in]
            n704 = Number To Decimal String(number="msinterval 5") -> (decimal integer string=w1545:string)  [unwired: 1 in]
            n705 = Number To Decimal String(number="flashnum 2") -> (decimal integer string=w1544:string)  [unwired: 1 in]
            n706 = Number To Decimal String(number="repeats  12") -> (decimal integer string=w1543:string)  [unwired: 1 in]
            n707 = Number To Decimal String(number="grayframes 2") -> (decimal integer string=w1533:string)  [unwired: 1 in]
            n708 = Number To Decimal String(number="flashbrightness 2") -> (decimal integer string=w1531:string)  [unwired: 1 in]
            n709 = call <vilib>:"Space Constant.vi"() -> ("String"=w1528:string)
            n710 = Multiply(x=w1538, y=100000.0) -> (x*y=w1536:dbl)
            n711 = To Long Integer(number=w1536) -> (32bit integer=w1539:i32)
            "seed  3" <- w1539
            n712 = Number To Decimal String(number="boxsize 2") -> (decimal integer string=w1530:string)  [unwired: 1 in]
            n713 = Number To Decimal String(number=w1539) -> (decimal integer string=w1535:string)  [unwired: 1 in]
            n714 = Number To Decimal String(number="xcenter 6") -> (decimal integer string=w1527:string)  [unwired: 1 in]
            n715 = Number To Decimal String(number="ycenter 6") -> (decimal integer string=w1524:string)  [unwired: 1 in]
            n716 = Concatenate Strings(w1550, w1528, w1547, w1528, w1546, w1528, w1545, w1528, w1544, w1528, w1543, w1528, w1535, w1528, w1533, w1528, w1531, w1528, w1530, w1528, w1527, w1528, w1524, w1528) -> (w1523:string)
          }
          frame "akmovingspots" {
            n717 = local read "number (0 to 1) 2"() -> (w1565:dbl)
            n718 = Number To Decimal String(number="pixels/frame") -> (decimal integer string=w1580:string)  [unwired: 1 in]
            n719 = Number To Decimal String(number=16) -> (decimal integer string=w1583:string)  [unwired: 1 in]
            n720 = Number To Decimal String(number="length") -> (decimal integer string=w1579:string)  [unwired: 1 in]
            n721 = Number To Decimal String(number="width") -> (decimal integer string=w1578:string)  [unwired: 1 in]
            n722 = Number To Decimal String(number="repeats 11") -> (decimal integer string=w1577:string)  [unwired: 1 in]
            n723 = Number To Decimal String(number="bardiv") -> (decimal integer string=w1571:string)  [unwired: 1 in]
            n724 = Number To Decimal String(number="barbrightness") -> (decimal integer string=w1559:string)  [unwired: 1 in]
            n725 = Number To Decimal String(number="backg 2") -> (decimal integer string=w1569:string)  [unwired: 1 in]
            n726 = call <vilib>:"Space Constant.vi"() -> ("String"=w1552:string)
            n727 = Multiply(x=w1565, y=100000.0) -> (x*y=w1567:dbl)
            n728 = To Long Integer(number=w1567) -> (32bit integer=w1566:i32)
            "seed" <- w1566
            n729 = Number To Decimal String(number="ycenter 5") -> (decimal integer string=w1553:string)  [unwired: 1 in]
            n730 = Number To Decimal String(number="xcenter 5") -> (decimal integer string=w1554:string)  [unwired: 1 in]
            n731 = Number To Decimal String(number="0 for 90, 1 for 45") -> (decimal integer string=w1562:string)  [unwired: 1 in]
            n732 = Number To Decimal String(number="graydelayframes") -> (decimal integer string=w1560:string)  [unwired: 1 in]
            n733 = Number To Decimal String(number="RFcentered=1") -> (decimal integer string=w1555:string)  [unwired: 1 in]
            n734 = Number To Decimal String(number=w1566) -> (decimal integer string=w1564:string)  [unwired: 1 in]
            n735 = Concatenate Strings(w1583, w1552, w1580, w1552, w1579, w1552, w1578, w1552, w1577, w1552, w1571, w1552, w1569, w1552, w1559, w1552, w1564, w1552, w1562, w1552, w1560, w1552, w1555, w1552, w1554, w1552, w1553, w1552) -> (w1573:string)
          }
          frame "akmovingspotsII" {
            n736 = local read "number (0 to 1) 2"() -> (w1599:dbl)
            n737 = Number To Decimal String(number="pixels/frame 3") -> (decimal integer string=w1613:string)  [unwired: 1 in]
            n738 = Number To Decimal String(number=27) -> (decimal integer string=w1616:string)  [unwired: 1 in]
            n739 = Number To Decimal String(number="length 3") -> (decimal integer string=w1612:string)  [unwired: 1 in]
            n740 = Number To Decimal String(number="width 3") -> (decimal integer string=w1611:string)  [unwired: 1 in]
            n741 = Number To Decimal String(number="repeats 16") -> (decimal integer string=w1610:string)  [unwired: 1 in]
            n742 = Number To Decimal String(number="bardiv 3") -> (decimal integer string=w1605:string)  [unwired: 1 in]
            n743 = Number To Decimal String(number="barbrightness 3") -> (decimal integer string=w1593:string)  [unwired: 1 in]
            n744 = Number To Decimal String(number="backg 4") -> (decimal integer string=w1603:string)  [unwired: 1 in]
            n745 = call <vilib>:"Space Constant.vi"() -> ("String"=w1586:string)
            n746 = Multiply(x=w1599, y=100000.0) -> (x*y=w1601:dbl)
            n747 = To Long Integer(number=w1601) -> (32bit integer=w1600:i32)
            "seed  6" <- w1600
            n748 = Number To Decimal String(number="ycenter 8") -> (decimal integer string=w1587:string)  [unwired: 1 in]
            n749 = Number To Decimal String(number="xcenter 8") -> (decimal integer string=w1588:string)  [unwired: 1 in]
            n750 = Number To Decimal String(number="0 for 90, 1 for 46") -> (decimal integer string=w1596:string)  [unwired: 1 in]
            n751 = Number To Decimal String(number="graydelayframes 3") -> (decimal integer string=w1594:string)  [unwired: 1 in]
            n752 = Number To Decimal String(number="RFcentered=1 2") -> (decimal integer string=w1589:string)  [unwired: 1 in]
            n753 = Number To Decimal String(number=w1600) -> (decimal integer string=w1598:string)  [unwired: 1 in]
            n754 = Concatenate Strings(w1616, w1586, w1613, w1586, w1612, w1586, w1611, w1586, w1610, w1586, w1605, w1586, w1603, w1586, w1593, w1586, w1598, w1586, w1596, w1586, w1594, w1586, w1589, w1586, w1588, w1586, w1587, w1586) -> (w1585:string)
          }
          frame "retinotopybars" {
            n755 = Number To Decimal String(number="bars") -> (decimal integer string=w1624:string)  [unwired: 1 in]
            n756 = Number To Decimal String(number="width 4") -> (decimal integer string=w1623:string)  [unwired: 1 in]
            n757 = Number To Decimal String(number="repeats 17") -> (decimal integer string=w1622:string)  [unwired: 1 in]
            n758 = Number To Decimal String(number="grayframes 3") -> (decimal integer string=w1619:string)  [unwired: 1 in]
            n759 = Number To Decimal String(number=28) -> (decimal integer string=w1625:string)  [unwired: 1 in]
            n760 = call <vilib>:"Space Constant.vi"() -> ("String"=w1620:string)
            n761 = Concatenate Strings(w1625, w1620, w1624, w1620, w1623, w1620, w1622, w1620, w1619) -> (w1618:string)
          }
          frame "slitGrtRand" {
            n762 = local read "number (0 to 1) 2"() -> (w1632:dbl)
            n763 = Number To Decimal String(number="bars  2") -> (decimal integer string=w1641:string)  [unwired: 1 in]
            n764 = Number To Decimal String(number="width  5") -> (decimal integer string=w1640:string)  [unwired: 1 in]
            n765 = Number To Decimal String(number="repeats  19") -> (decimal integer string=w1639:string)  [unwired: 1 in]
            n766 = Number To Decimal String(number="grayframes  4") -> (decimal integer string=w1637:string)  [unwired: 1 in]
            n767 = Multiply(x=w1632, y=100000.0) -> (x*y=w1634:dbl)
            n768 = Number To Decimal String(number=32) -> (decimal integer string=w1642:string)  [unwired: 1 in]
            n769 = call <vilib>:"Space Constant.vi"() -> ("String"=w1631:string)
            n770 = To Long Integer(number=w1634) -> (32bit integer=w1633:i32)
            "seed 4" <- w1633
            n771 = Number To Decimal String(number=w1633) -> (decimal integer string=w1630:string)  [unwired: 1 in]
            n772 = Concatenate Strings(w1642, w1631, w1641, w1631, w1640, w1631, w1639, w1631, w1637, w1631, w1630) -> (w1636:string)
          }
          frame "slitGrtOrder" {
            n773 = local read "number (0 to 1) 2"() -> (w1650:dbl)
            n774 = Number To Decimal String(number="bars  3") -> (decimal integer string=w1658:string)  [unwired: 1 in]
            n775 = Number To Decimal String(number="width  6") -> (decimal integer string=w1657:string)  [unwired: 1 in]
            n776 = Number To Decimal String(number="repeats  20") -> (decimal integer string=w1656:string)  [unwired: 1 in]
            n777 = Number To Decimal String(number="grayframes  5") -> (decimal integer string=w1654:string)  [unwired: 1 in]
            n778 = Multiply(x=w1650, y=100000.0) -> (x*y=w1652:dbl)
            n779 = Number To Decimal String(number=34) -> (decimal integer string=w1659:string)  [unwired: 1 in]
            n780 = call <vilib>:"Space Constant.vi"() -> ("String"=w1649:string)
            n781 = To Long Integer(number=w1652) -> (32bit integer=w1651:i32)
            "seed 5" <- w1651
            n782 = Number To Decimal String(number=w1651) -> (decimal integer string=w1648:string)  [unwired: 1 in]
            n783 = Concatenate Strings(w1659, w1649, w1658, w1649, w1657, w1649, w1656, w1649, w1654, w1649, w1648) -> (w1647:string)
          }
          frame "singledirection" {
            n784 = local read "number (0 to 1) 2"() -> (w1672:dbl)
            n785 = Number To Decimal String(number="pixels/frame 2") -> (decimal integer string=w1686:string)  [unwired: 1 in]
            n786 = Number To Decimal String(number=22) -> (decimal integer string=w1689:string)  [unwired: 1 in]
            n787 = Number To Decimal String(number="length 2") -> (decimal integer string=w1685:string)  [unwired: 1 in]
            n788 = Number To Decimal String(number="width 2") -> (decimal integer string=w1684:string)  [unwired: 1 in]
            n789 = Number To Decimal String(number="repeats 12") -> (decimal integer string=w1683:string)  [unwired: 1 in]
            n790 = Number To Decimal String(number="bardiv 2") -> (decimal integer string=w1678:string)  [unwired: 1 in]
            n791 = Number To Decimal String(number="barbrightness 2") -> (decimal integer string=w1667:string)  [unwired: 1 in]
            n792 = Number To Decimal String(number="backg 3") -> (decimal integer string=w1676:string)  [unwired: 1 in]
            n793 = call <vilib>:"Space Constant.vi"() -> ("String"=w1670:string)
            n794 = Multiply(x=w1672, y=100000.0) -> (x*y=w1674:dbl)
            n795 = To Long Integer(number=w1674) -> (32bit integer=w1673:i32)
            "seed  4" <- w1673
            n796 = Number To Decimal String(number="degrees") -> (decimal integer string=w1668:string)  [unwired: 1 in]
            n797 = Number To Decimal String(number="graydelayframes 2") -> (decimal integer string=w1665:string)  [unwired: 1 in]
            n798 = Number To Decimal String(number=w1673) -> (decimal integer string=w1671:string)  [unwired: 1 in]
            n799 = Concatenate Strings(w1689, w1670, w1686, w1670, w1685, w1670, w1684, w1670, w1683, w1670, w1678, w1670, w1676, w1670, w1667, w1670, w1671, w1670, w1668, w1670, w1665, w1667) -> (w1664:string)
          }
          frame "randgrat" {
            n800 = local read "number (0 to 1) 2"() -> (w1691:dbl)
            n801 = Number To Decimal String(number="cycles per second 3") -> (decimal integer string=w1705:string)  [unwired: 1 in]
            n802 = Number To Decimal String(number=12) -> (decimal integer string=w1708:string)  [unwired: 1 in]
            n803 = Multiply(x=w1691, y=100000.0) -> (x*y=w1695:dbl)
            n804 = Number To Decimal String(number="period 3") -> (decimal integer string=w1704:string)  [unwired: 1 in]
            n805 = Number To Decimal String(number="duration 3") -> (decimal integer string=w1703:string)  [unwired: 1 in]
            n806 = Number To Decimal String(number="repeats 13") -> (decimal integer string=w1702:string)  [unwired: 1 in]
            n807 = Number To Decimal String(number="amplitude 3") -> (decimal integer string=w1701:string)  [unwired: 1 in]
            n808 = call <vilib>:"Space Constant.vi"() -> ("String"=w1693:string)
            n809 = To Long Integer(number=w1695) -> (32bit integer=w1692:i32)
            "seed 2" <- w1692
            n810 = Number To Decimal String(number=w1692) -> (decimal integer string=w1694:string)  [unwired: 1 in]
            n811 = Concatenate Strings(w1708, w1693, w1705, w1693, w1704, w1693, w1703, w1693, w1702, w1693, w1701, w1693, w1694, w1693) -> (w1697:string)
          }
          frame "squarewave" {
            n812 = local read "number (0 to 1) 2"() -> (w1711:dbl)
            n813 = Number To Decimal String(number="cycles per second 4") -> (decimal integer string=w1724:string)  [unwired: 1 in]
            n814 = Number To Decimal String(number=31) -> (decimal integer string=w1727:string)  [unwired: 1 in]
            n815 = Multiply(x=w1711, y=100000.0) -> (x*y=w1715:dbl)
            n816 = Number To Decimal String(number="period 4") -> (decimal integer string=w1723:string)  [unwired: 1 in]
            n817 = Number To Decimal String(number="duration 5") -> (decimal integer string=w1722:string)  [unwired: 1 in]
            n818 = Number To Decimal String(number="repeats 14") -> (decimal integer string=w1721:string)  [unwired: 1 in]
            n819 = Number To Decimal String(number="amplitude 4") -> (decimal integer string=w1720:string)  [unwired: 1 in]
            n820 = call <vilib>:"Space Constant.vi"() -> ("String"=w1713:string)
            n821 = To Long Integer(number=w1715) -> (32bit integer=w1712:i32)
            "seed 3" <- w1712
            n822 = Number To Decimal String(number=w1712) -> (decimal integer string=w1714:string)  [unwired: 1 in]
            n823 = Concatenate Strings(w1727, w1713, w1724, w1713, w1723, w1713, w1722, w1713, w1721, w1713, w1720, w1713, w1714, w1713) -> (w1710:string)
          }
          frame "LatCrinkleMultAlt" {
            n824 = Number To Decimal String(number="Loops") -> (decimal integer string=w1731:string)  [unwired: 1 in]
            n825 = Number To Decimal String(number="waitForDeviceStart") -> (decimal integer string=w1739:string)  [unwired: 1 in]
            n826 = Number To Decimal String(number="startCue") -> (decimal integer string=w1740:string)  [unwired: 1 in]
            n827 = Number To Decimal String(number="Repeats") -> (decimal integer string=w1743:string)  [unwired: 1 in]
            n828 = Number To Decimal String(number="beepPauseTime") -> (decimal integer string=w1741:string)  [unwired: 1 in]
            n829 = Number To Decimal String(number="beepLengthSecs") -> (decimal integer string=w1742:string)  [unwired: 1 in]
            n830 = Number To Decimal String(number="Frequency") -> (decimal integer string=w1744:string)  [unwired: 1 in]
            n831 = Number To Decimal String(number=37) -> (decimal integer string=w1745:string)  [unwired: 1 in]
            n832 = call <vilib>:"Space Constant.vi"() -> ("String"=w1730:string)
            n833 = Concatenate Strings(w1745, w1730, w1744, w1730, w1743, w1730, w1742, w1730, w1741, w1730, w1740, w1730, w1739, w1730, w1731, w1730) -> (w1729:string)
          }
          frame "LatCrinkleOneAlt" {
            n834 = Number To Decimal String(number="waitForDeviceStart  2") -> (decimal integer string=w1754:string)  [unwired: 1 in]
            n835 = Number To Decimal String(number="startCue 2") -> (decimal integer string=w1755:string)  [unwired: 1 in]
            n836 = Number To Decimal String(number="Repeats 2") -> (decimal integer string=w1759:string)  [unwired: 1 in]
            n837 = Number To Decimal String(number="beepPauseTime 2") -> (decimal integer string=w1757:string)  [unwired: 1 in]
            n838 = Number To Decimal String(number="beepLengthSecs 2") -> (decimal integer string=w1758:string)  [unwired: 1 in]
            n839 = Number To Decimal String(number="Frequency 2") -> (decimal integer string=w1760:string)  [unwired: 1 in]
            n840 = Number To Decimal String(number=36) -> (decimal integer string=w1761:string)  [unwired: 1 in]
            n841 = call <vilib>:"Space Constant.vi"() -> ("String"=w1756:string)
            n842 = Concatenate Strings(w1761, w1756, w1760, w1756, w1759, w1756, w1758, w1756, w1757, w1756, w1755, w1756, w1754, w1756) -> (w1747:string)
          }
          frame "SqrGrtPtch" {
            n843 = local read "number (0 to 1) 2"() -> (w1773:dbl)
            n844 = Number To Decimal String(number="appatchsizelitude 6") -> (decimal integer string=w1766:string)  [unwired: 1 in]
            n845 = Number To Decimal String(number="xcenter 9") -> (decimal integer string=w1768:string)  [unwired: 1 in]
            n846 = Number To Decimal String(number="ycenter 7") -> (decimal integer string=w1767:string)  [unwired: 1 in]
            n847 = Number To Decimal String(number="cycles per second 5") -> (decimal integer string=w1785:string)  [unwired: 1 in]
            n848 = Number To Decimal String(number=26) -> (decimal integer string=w1788:string)  [unwired: 1 in]
            n849 = Multiply(x=w1773, y=100000.0) -> (x*y=w1776:dbl)
            n850 = Number To Decimal String(number="period 5") -> (decimal integer string=w1784:string)  [unwired: 1 in]
            n851 = Number To Decimal String(number="duration 6") -> (decimal integer string=w1783:string)  [unwired: 1 in]
            n852 = Number To Decimal String(number="repeats 15") -> (decimal integer string=w1782:string)  [unwired: 1 in]
            n853 = Number To Decimal String(number="amplitude 5") -> (decimal integer string=w1781:string)  [unwired: 1 in]
            n854 = call <vilib>:"Space Constant.vi"() -> ("String"=w1764:string)
            n855 = To Long Integer(number=w1776) -> (32bit integer=w1774:i32)
            "seed 6" <- w1774
            n856 = Number To Decimal String(number=w1774) -> (decimal integer string=w1775:string)  [unwired: 1 in]
            n857 = Number To Decimal String(number="xcenter 7") -> (decimal integer string=w1763:string)  [unwired: 1 in]
            n858 = Concatenate Strings(w1788, w1764, w1785, w1764, w1784, w1764, w1783, w1764, w1782, w1764, w1781, w1764, w1775, w1764, w1768, w1764, w1767, w1764, w1766, w1764, w1763, w1764) -> (w1772:string)
          }
          frame "SqrGrtPtch 2" {
            n859 = local read "number (0 to 1) 2"() -> (w1800:dbl)
            n860 = Number To Decimal String(number="asdf") -> (decimal integer string=w1794:string)  [unwired: 1 in]
            n861 = Number To Decimal String(number="numpatches") -> (decimal integer string=w1796:string)  [unwired: 1 in]
            n862 = Number To Decimal String(number="asdf 2") -> (decimal integer string=w1795:string)  [unwired: 1 in]
            n863 = Number To Decimal String(number="cycles per second 6") -> (decimal integer string=w1812:string)  [unwired: 1 in]
            n864 = Number To Decimal String(number=33) -> (decimal integer string=w1815:string)  [unwired: 1 in]
            n865 = Multiply(x=w1800, y=100000.0) -> (x*y=w1803:dbl)
            n866 = Number To Decimal String(number="period 6") -> (decimal integer string=w1811:string)  [unwired: 1 in]
            n867 = Number To Decimal String(number="duration 7") -> (decimal integer string=w1810:string)  [unwired: 1 in]
            n868 = Number To Decimal String(number="repeats 19") -> (decimal integer string=w1809:string)  [unwired: 1 in]
            n869 = Number To Decimal String(number="amplitude 6") -> (decimal integer string=w1808:string)  [unwired: 1 in]
            n870 = call <vilib>:"Space Constant.vi"() -> ("String"=w1792:string)
            n871 = To Long Integer(number=w1803) -> (32bit integer=w1801:i32)
            "seed 7" <- w1801
            n872 = Number To Decimal String(number=w1801) -> (decimal integer string=w1802:string)  [unwired: 1 in]
            n873 = Number To Decimal String(number="xcenter 10") -> (decimal integer string=w1791:string)  [unwired: 1 in]
            n874 = Concatenate Strings(w1815, w1792, w1812, w1792, w1811, w1792, w1810, w1792, w1809, w1792, w1808, w1792, w1802, w1792, w1796, w1792, w1795, w1792, w1794, w1792, w1791, w1792) -> (w1790:string)
          }
          frame "Fullfield" {
            # "The stim info ref goes nowhere? \nWhere should we save this text file?"
            # "Where are the coord numbers coming from?"
            n875 = Number To Decimal String(number="# of flashes 2") -> (decimal integer string=w1819:string)  [unwired: 1 in]
            n876 = Number To Decimal String(number=8) -> (decimal integer string=w1822:string)  [unwired: 1 in]
            n877 = Number To Decimal String(number="flash frame length 2") -> (decimal integer string=w1818:string)  [unwired: 1 in]
            n878 = call <vilib>:"Space Constant.vi"() -> ("String"=w1817:string)
            n879 = Concatenate Strings(w1822, w1817, w1819, w1817, w1818) -> (w1823:string)
          }
        }
        n880 = event shown="[1] \"Start Stimulus\": Value Change" {
          selector: _ -> [_ _]
          dyn-events: _ -> [_ _]
          timeout: 1000 -> [_ _]
          tunnel: [w1825 w1832] -> w1190
          tunnel: w1175 -> [_ w1830]
          tunnel: [_ w1829] -> w1174
          event Timeout {
            n881 = event-data() -> ()  [unwired: 1 in, 2 out]
            n882 = Concatenate Strings("9" ("string"), "\r\n", "") -> (w1825:string)
          }
          event "Start Stimulus": Value Change {
            n883 = event-data() -> ("NewVal"=w1831:bool)  [unwired: 1 in, 4 out]
            n884 = case shown="True" w1831 {
              tunnel: ["" w1839] -> w1832
              tunnel: w1830 -> [_ w1836]
              tunnel: [_ w1835] -> w1829
              frame False {
              }
              frame True {
                n885 = local read "File Open"() -> (w1834:bool)
                n886 = case shown="False" w1834 {
                  tunnel: [w1842 w1850] -> w1837
                  tunnel: [w1842 _] -> w1835
                  frame False {
                    n887 = Temporary Directory() -> (w1846:path)
                    n888 = Path To String(path=w1846) -> (string=w1845:string)
                    n889 = Concatenate Strings(w1845, "Stimtemp" ("string"), ".txt" ("string")) -> (w1844:string)
                    n890 = String To Path(string=w1844) -> (path=w1843:path)
                    n891 = Open/Create/Replace File(file path (use dialog)=w1843, operation (0:open)=T9."replace or create") -> (refnum out=w1842:refnum<file>)  [unwired: 1 in, 5 out]
                  }
                  frame True {
                    n892 = local read "Stim ref out"() -> (w1850:refnum<file>)
                  }
                }
                n893 = Write to Text File(file (use dialog)=w1837, text=w1836) -> (refnum out=→"Stim ref out 2":refnum<file>)  [unwired: 2 in, 2 out]
                n894 = Concatenate Strings(w1836, "\r\n", "") -> (w1839:string)
              }
            }
          }
        }
        n895 = call <vilib>:"Space Constant.vi"() -> ("String"=w1181:string)
        n896 = Multiply(x="frames to avg", y=w1185) -> (x*y=w1186:i32)
        n897 = Number To Decimal String(number=w1186, width (-)=6) -> (decimal integer string=w1187:string)
        n898 = Number To Decimal String(number=w1185, width (-)=3) -> (decimal integer string=w1184:string)
        n899 = Concatenate Strings(w1182, w1181, w1187, w1181, w1184, w1181) -> (→"Input Line":string)
        n900 = Concatenate Strings(w1196, w1190) -> (w1194:string)
        n901 = case shown="False" "Stop TCP Write" {
          tunnel: w1190 -> [w1852 _]
          tunnel: [w1851 w1854] -> w1192
          tunnel: w1193 -> [w1853 _]
          frame False {
            n902 = TCP Write(connection ID=w1853, data in=w1852) -> (error out=w1851:errorcluster)  [unwired: 2 in, 2 out]
          }
          frame True {
            n903 = call <vilib>:"Clear Errors.vi"() -> ("error out"=w1854:errorcluster)  [unwired: 6 in, 1 out]
          }
        }
        n904 = Unbundle By Name(w1192) -> ("status"=w1191:bool)
        n905 = Or(x=w1191, y="Stop TCP Write") -> (x .or. y?=w1195:bool)
        "TCP Loop\nRunning" <- TRUE
      }
      "TCP Listen\nStopped" <- w1163
      n906 = Flush File(refnum=w1162) -> ()  [unwired: 1 in, 2 out]
      n907 = Build Array(w1171) -> (w1164:errorcluster[])
      n908 = Merge Errors(w1164) -> (w1170:errorcluster)
      n909 = call <vilib>:"Error to Warning.vi"("1st Error to Convert"=w1169, "2nd Error to Convert"=w1166, "3rd Error to Convert"=w1168, "error in"=w1170) -> ("warning out"=w1167:errorcluster)  [unwired: 11 in]
    }
    frame Error {
    }
  }
  n910 = node-c288(w26) -> ()  [unwired: 1 out]
  n911 = UDP Close(connection ID=w29, 8:w28) -> ()  [unwired: 2 out]
  n912 = flat-sequence {
    frame #0 {
      w1858 = FALSE ("File Open")
      n913 = local write "TCP Loop\nRunning"(w1858) -> ()
      n914 = local write "Save Time Start"(w1858) -> ()
      n915 = local write "File Open"(w1858) -> ()
      n916 = local write "Correct"(w1858) -> ()
      n917 = property on="SAVE" class="Bool (strict)"("Val(Sgnl)"=w1858) -> ()  [unwired: 2 in, 2 out]
    }
    frame #1 {
      n918 = while {
        shift-right: [w1861] -> _
        shift-left: 0 ("number") -> [w1862]
        stop <- "Close Save" stop-if-true
        n919 = event shown="[1] \"SAVE\": Value Change" {
          selector: _ -> [_ _]
          dyn-events: _ -> [_ _]
          timeout: -1 -> [_ _]
          tunnel: w1862 -> [w1864 w1867]
          tunnel: [w1864 w1866] -> w1861
          event Timeout {
            n920 = event-data() -> ()  [unwired: 1 in, 3 out]
          }
          event "SAVE": Value Change {
            n921 = event-data() -> ()  [unwired: 1 in, 6 out]
            n922 = property on="SAVE" class="Bool (strict)"() -> ("Value"=w1865:bool)  [unwired: 2 in, 2 out]
            n923 = case shown="True" w1865 {
              tunnel: w1867 -> [w1869 w1880]
              tunnel: [w1869 w1879] -> w1866
              frame False {
                n924 = local read "File Open"() -> (w1868:bool)
                n925 = case shown="True" w1868 {
                  frame False {
                  }
                  frame True {
                    n926 = stacked-sequence {
                      frame #0 {
                        n927 = local write "File Open"(FALSE ("Movie Open")) -> ()
                      }
                      frame #1 {
                        n928 = Wait (ms)(milliseconds to wait=u32 20) -> ()  [unwired: 1 out]
                      }
                      frame #2 {
                        n929 = local read "TCP Loop\nRunning"() -> (w1876:bool)
                        n930 = local read "Encoder\n Ref Out 2"() -> (w1873:refnum<file>)
                        n931 = case shown="True" w1876 {
                          frame False {
                          }
                          frame True {
                            n932 = local read "Stim ref out 2"() -> (w1877:refnum<file>)
                            n933 = Close File(refnum=w1877) -> ()  [unwired: 1 in, 2 out]
                          }
                        }
                        n934 = local read "PCO Ref Out 2"() -> (w1875:refnum<file>)
                        n935 = Close File(refnum=w1873) -> (error out=→"Encoder Ref Error":errorcluster)  [unwired: 1 in, 1 out]
                        n936 = Close File(refnum=w1875) -> (error out=→"PCo Ref Error":errorcluster)  [unwired: 1 in, 1 out]
                      }
                    }
                  }
                }
              }
              frame True {
                n937 = local read "File Open"() -> (w1878:bool)
                n938 = case shown="False" w1878 {
                  tunnel: w1880 -> [w1881 w1909]
                  tunnel: [w1907 w1909] -> w1879
                  frame False {
                    n939 = local read "File Save Path"() -> (w1883:path)
                    n940 = Increment(x=w1881) -> (x+1=w1907:i32)
                    "File Iterations" <- w1907
                    n941 = Number To Decimal String(number=w1881) -> (decimal integer string=w1897:string)  [unwired: 1 in]
                    n942 = Path To String(path=w1883) -> (string=w1906:string)
                    n943 = Path To String(path=w1883) -> (string=w1902:string)
                    n944 = Concatenate Strings(w1906, "\\" ("string"), "_stim" ("string"), w1897, ".txt" ("string")) -> (w1891:string)
                    n945 = Concatenate Strings(w1902, "\\" ("string"), w1897, "2Pmov.dat" ("string")) -> (w1901:string)
                    n946 = Number To Decimal String(number=w1881) -> (decimal integer string=w1890:string)  [unwired: 1 in]
                    n947 = String To Path(string=w1901) -> (path=w1899:path)
                    n948 = Path To String(path=w1883) -> (string=w1885:string)
                    n949 = Open/Create/Replace File(file path (use dialog)=w1899, operation (0:open)=T9."create") -> (refnum out=w1893:refnum<file>)  [unwired: 4 in, 2 out]
                    "PCO ref out" <- w1893
                    n950 = Concatenate Strings(w1885, "\\" ("string"), w1890, "Licks&Position.dat" ("string")) -> (w1886:string)
                    n951 = String To Path(string=w1891) -> (path=w1896:path)
                    n952 = String To Path(string=w1886) -> (path=w1888:path)
                    n953 = stacked-sequence {
                      tunnel: w1893 -> [_]
                      frame #0 {
                        "File Open" <- TRUE ("Close All")
                      }
                    }
                    n954 = Open/Create/Replace File(file path (use dialog)=w1896, operation (0:open)=T9."create") -> (refnum out=→"Stim ref out":refnum<file>)  [unwired: 1 in, 5 out]
                    n955 = Open/Create/Replace File(file path (use dialog)=w1888, operation (0:open)=T9."create") -> (refnum out=→"Encoder Ref Out":refnum<file>)  [unwired: 4 in, 2 out]
                  }
                  frame True {
                  }
                }
              }
            }
          }
        }
      }
    }
  }
  n956 = local write "TCP Listen\nStopped"(w105) -> ()
  n957 = TCP Close Connection(connection ID=w107, error in (no error)=w106) -> ()  [unwired: 1 in, 2 out]
